vi "MEDIDA_cRIO_ZNB_AMI.vi"(8 "error in (no error)":errorcluster) -> (0 "error out":errorcluster)   [LabVIEW 2017]
uses:
  MEDIDA_cRIO_ZNB_AMI_DATOS.ctl
  MEDIDA_cRIO_ZNB_AMI.ctl
  RohdeSchwarz ZNB MeasConfig.ctl
  AMI MAGNET/Status AMI.ctl
  DISPLAY/Display_Command Control.ctl
  DISPLAY/DataType.ctl
  TIMING/Timing_Module Control.ctl
  cRIO_ZNB_AMI_GLOBALES.vi
  FILE/File_Module Control.ctl
  <instrlib>/Agilent ENA Series/Agilent ENA Series.lvlib
panel:
  out "Z.Stable":bool
  out "Y.Stable":bool
  out "X.Stable":bool
  out "wZ.Stable":bool
  out "wY.Stable":bool
  out "wX.Stable":bool
  out "Z.WaitStability":bool
  out "Y.WaitStability":bool
  out "X.WaitStability":bool
  out "X state":T1=1 items=["Unknown", "RAMPING to target field/current", "HOLDING at the target field/current", "PAUSED", "Ramping in MANUAL UP mode", "Ramping in MANUAL DOWN mode", "ZEROING CURRENT (in progress)", "Quench detected", "At ZERO current", "Heating persistent switch", "Cooling persistent switch", "External Rampdown active"]
  out "Y state":T1=1 items=["Unknown", "RAMPING to target field/current", "HOLDING at the target field/current", "PAUSED", "Ramping in MANUAL UP mode", "Ramping in MANUAL DOWN mode", "ZEROING CURRENT (in progress)", "Quench detected", "At ZERO current", "Heating persistent switch", "Cooling persistent switch", "External Rampdown active"]
  out "Z state":T1=1 items=["Unknown", "RAMPING to target field/current", "HOLDING at the target field/current", "PAUSED", "Ramping in MANUAL UP mode", "Ramping in MANUAL DOWN mode", "ZEROING CURRENT (in progress)", "Quench detected", "At ZERO current", "Heating persistent switch", "Cooling persistent switch", "External Rampdown active"]
  out "Z Modo Rampa":u16(ring)=1 items=["RAMP", "PAUSE", "PAUSE", "MANUAL DOWN", "ZERO"]
  out "Z Rate":dbl
  out "Z Field":dbl
  out "Y Modo Rampa":u16(ring)=1 items=["RAMP", "PAUSE", "PAUSE", "MANUAL DOWN", "ZERO"]
  out "Y Rate":dbl
  out "Y Field":dbl
  out "X Modo Rampa":u16(ring)=1 items=["RAMP", "PAUSE", "PAUSE", "MANUAL DOWN", "ZERO"]
  out "X Rate":dbl
  out "X Field":dbl
  in  "ID Query? (T: Yes)":bool=TRUE
  in  "Reset? (T: Yes)":bool
  out "XY lastMeas":cluster{dbl[], dbl[]}(graph)
  in  "VISA resource":refnum<visa-resource-name>="ZNB20-62-101710"
  out "ENA3G path":path caption="selected path"
  out "MeasConfig":T2={"Tiempo (sec)"=10.0, "Campo X (T)"=0.025, "Campo Y (T)"=10.0, "Campo Z (T)"=0.025, "Temperatura (K)"=0.025, "Start Frequency (Hz)"=100000.0, "Stop Frequency (Hz)"=1000000.0, "IF Bandwidth"=25.0, "Sweep time(s)"=25.0, "Meas Points"=201, "Power Level (0.0)"=-40.0} {"Campo Z (T)" format="%^.2e"; "Campo Y (T)" format="%^.2e"; "Sweep time(s)" format="%^.2g"; "Temperatura (K)" format="%^.2e"; "Campo X (T)" format="%^.2e"; "Tiempo (sec)" format="%^.2g"; "Start Frequency (Hz)" format="%^.2e"; "IF Bandwidth" format="%^.2e"; "Power Level (0.0)" format="%^.2g"}
  out "Voltage Status":i32(ring) items=["VoltageUnknown", "Stable", "Tracking"]
  out "wV.Stable":bool
  out "V.Stable":bool
  out "V.WaitStability":bool
  out "Command":T3
  out "T.Stable":bool
  out "#seconds":dbl=300.0
  out "currentPoint":i16=300
  out "dSeconds":dbl=300.0
  out "averages":i16=300
  out "#points":i16=300
  out "On timeout":i32(ring) items=["Continue", "Abort "]
  out "StabilityTimeout(s)":dbl=300.0
  out "wT.Stable":bool
  out "T.WaitStability":bool
  out "#IntruccionActual":i32
  out "#Intrucciones":i32
  out "Temperature Status":i32(ring) items=["TemperatureUnknown", "Stable", "Tracking", "Near"]
  out "cRIO Stable":bool
  out "Datos":T4 {"CampoZ(T)" format="%.3e"; "CampoY(T)" format="%.3e"; "A.Input3(V)" format="%.3e"; "A.Input4(V)" format="%.3e"; "A.Input1(V)" format="%.3e"; "A.Input2(V)" format="%.3e"; "Temperatura(K)" format="%.3e"; "CampoX(T)" format="%.3e"; "Tiempo(min)" format="%.3e"}
  # "cRIO"
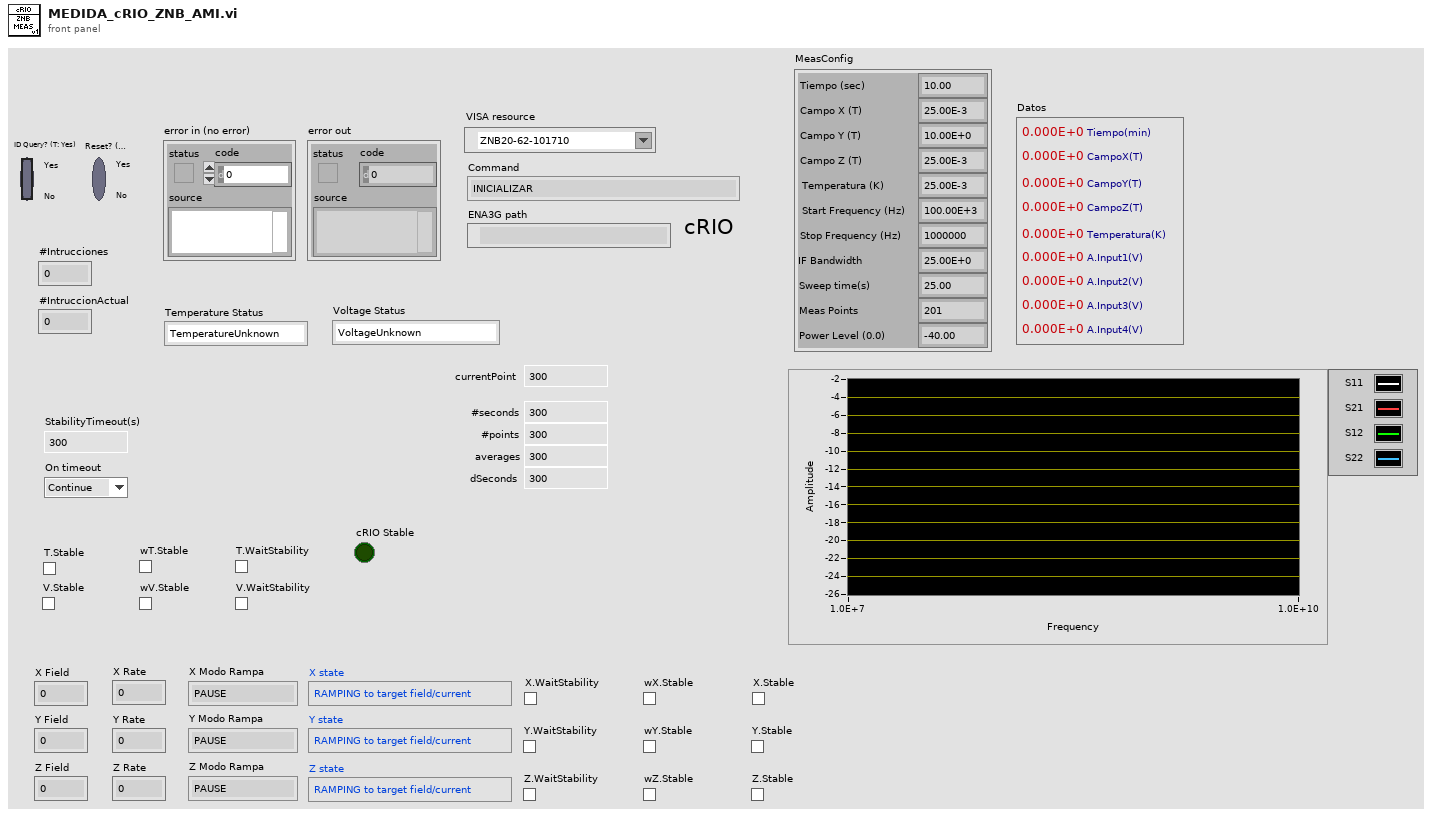
[diagram p1: front panel]
types:
  T1 = typedef "Status AMI.ctl" = u16
  T2 = typedef "RohdeSchwarz ZNB MeasConfig.ctl" = cluster{"Tiempo (sec)":dbl, "Campo X (T)":dbl, "Campo Y (T)":dbl, "Campo Z (T)":dbl, "Temperatura (K)":dbl, "Start Frequency (Hz)":dbl, "Stop Frequency (Hz)":dbl, "IF Bandwidth":dbl, "Sweep time(s)":dbl, "Meas Points":i32, "Power Level (0.0)":dbl}
  T3 = typedef "MEDIDA_cRIO_ZNB_AMI.ctl" = enum16{"INICIALIZAR", "TEST COMMAND", "SET FIELD X", "LOOK STABLE FIELD X", "SET FIELD Y", "LOOK STABLE FIELD Y", "SET FIELD Z", "LOOK STABLE FIELD Z", "SET TEMPERATURE", "LOOK STABLE TEMPERATURE", "SET VOLTAGE", "LOOK STABLE VOLTAGE", "WAIT PARAMETERS", "LOOK STABILITY", "MEASURE PARAMETERS", "SCAN READ TIME, B y T", "SCAN READ cRIO", "MEASURE SWEEP", "SWEEP READ TIME, B y T", "SWEEP READ cRIO", "MEASURE ENA3G / ZNB", "PAUSE SEQUENCE", "FINALIZAR"}
  T4 = typedef "MEDIDA_cRIO_ZNB_AMI_DATOS.ctl" = cluster{"Tiempo(min)":dbl, "CampoX(T)":dbl, "CampoY(T)":dbl, "CampoZ(T)":dbl, "Temperatura(K)":dbl, "A.Input1(V)":dbl, "A.Input2(V)":dbl, "A.Input3(V)":dbl, "A.Input4(V)":dbl}
  T5 = typedef "DataType.ctl" = enum16{"Initialize Front Panel", "Update Front Panel", "Update Graph", "Enable/Disable Controls", "Update Status"}
  T6 = typedef "Display_Command Control.ctl" = enum16{"Initialize", "Generate Event", "Shutdown"}
  T7 = enum16{"open", "replace", "create", "open or create", "replace or create", "replace or create with confirmation"}
  T8 = typedef "Timing_Module Control.ctl" = enum16{"Initialize Time", "Check Time"}
  T9 = typedef "File_Module Control.ctl" = enum16{"Initialize", "Save Head", "Save Data", "Shutdown"}
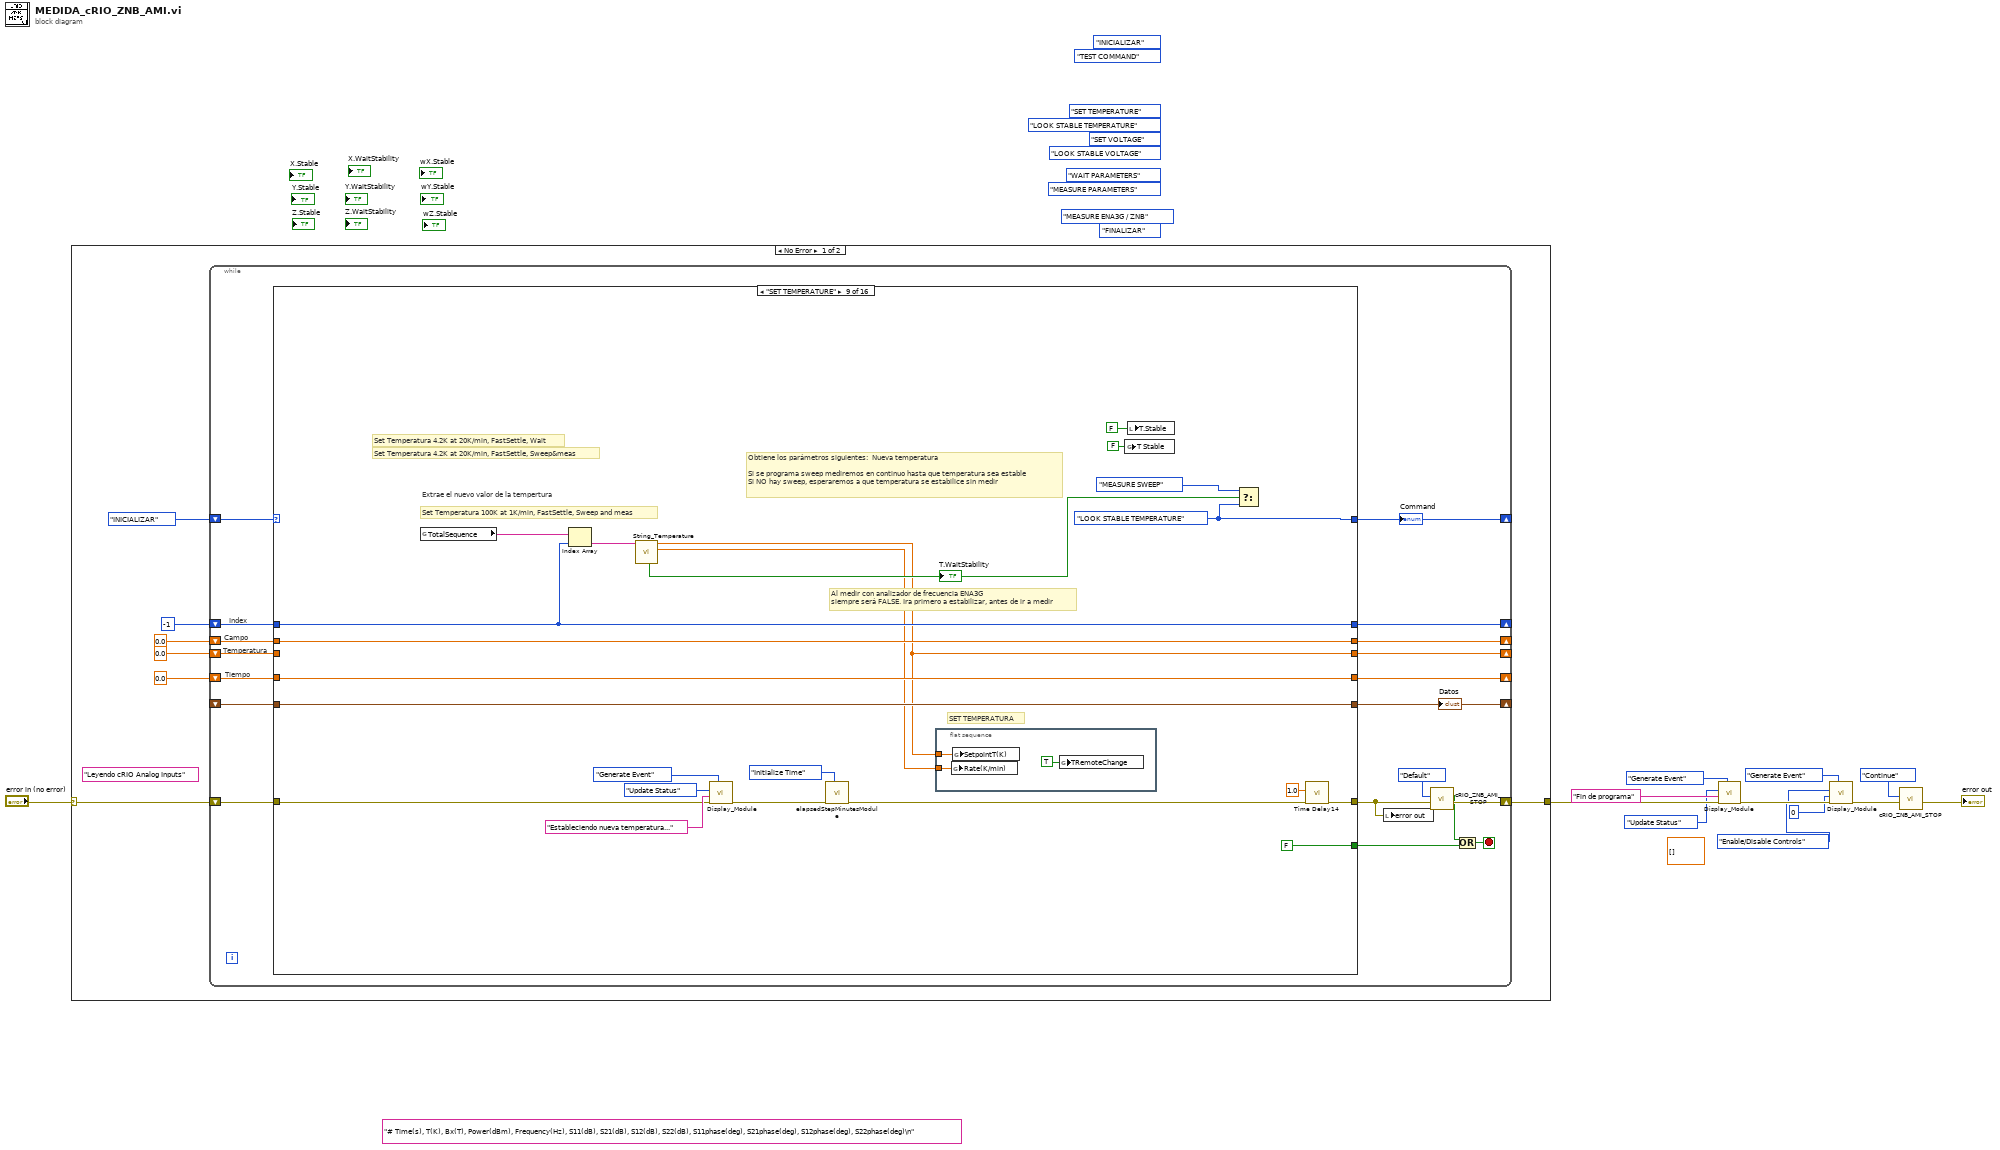
[diagram p0: block diagram]
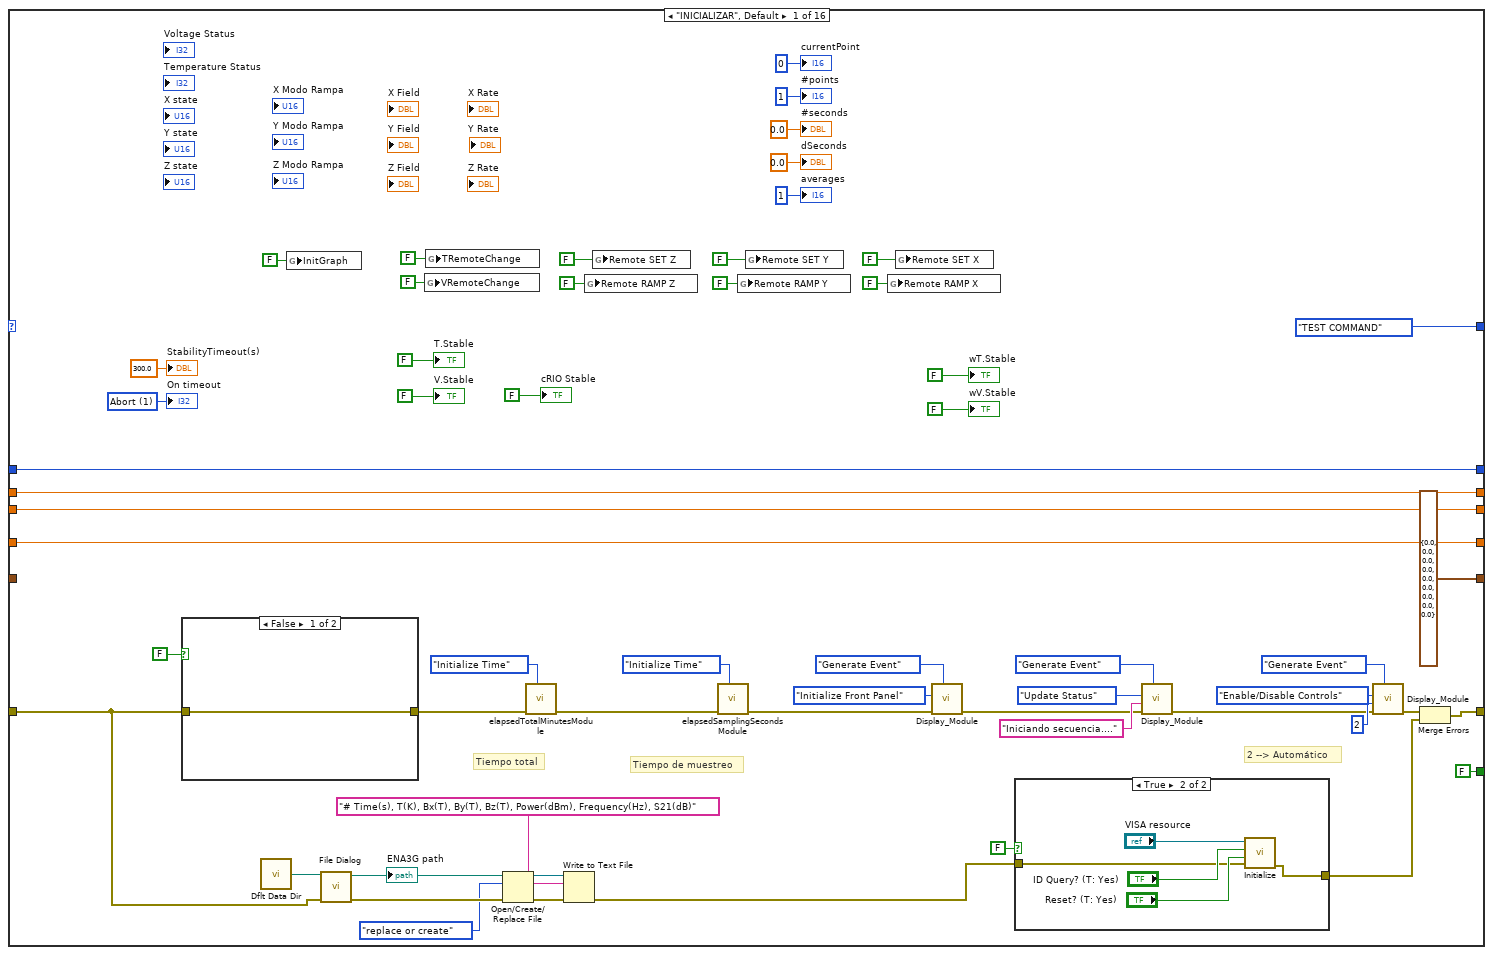
[diagram p2: hidden frame]
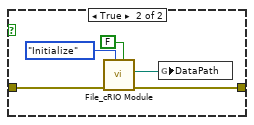
[diagram p4: hidden frame]
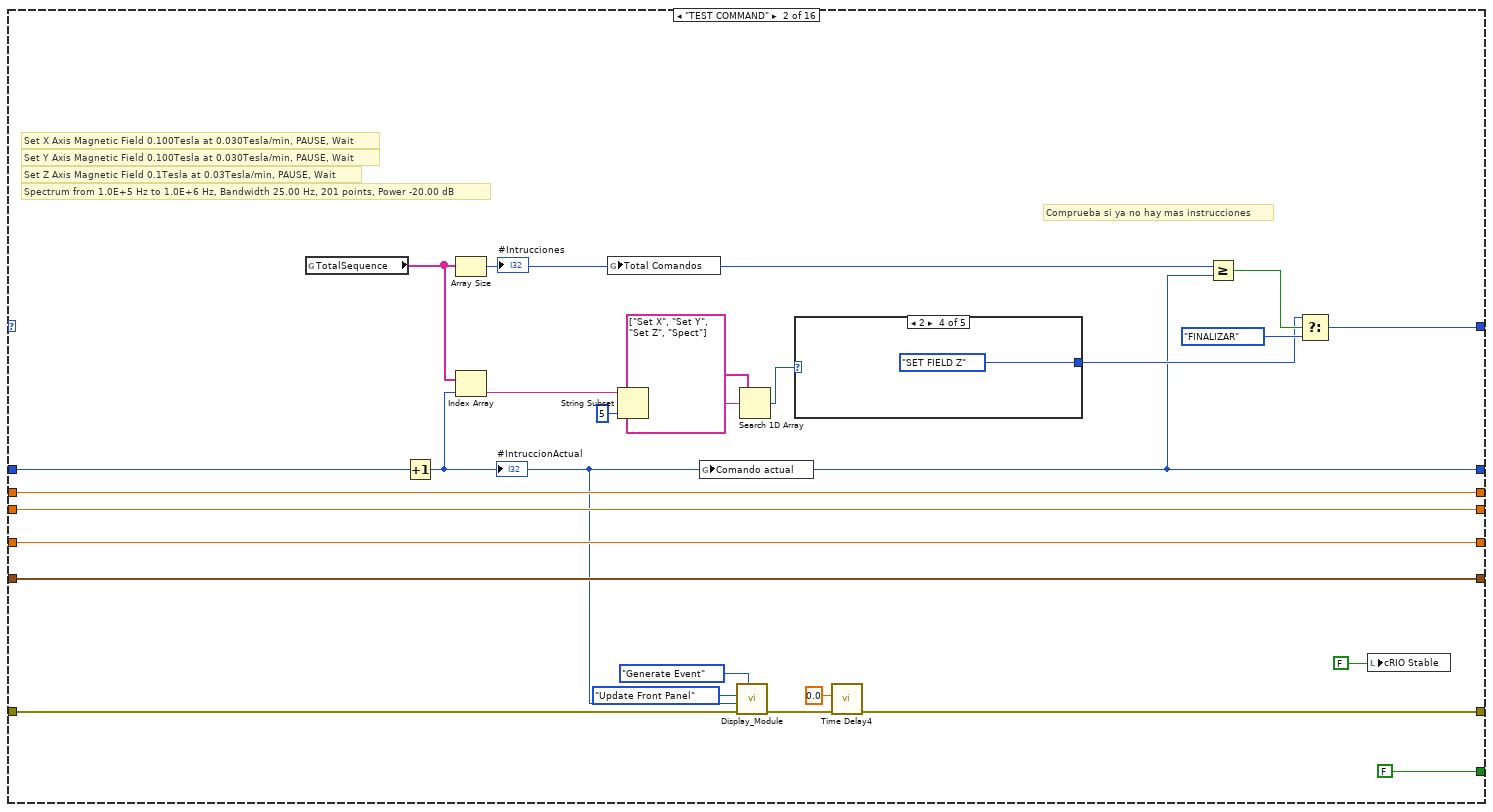
[diagram p5: hidden frame]
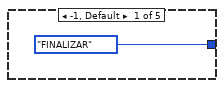
[diagram p6: hidden frame]
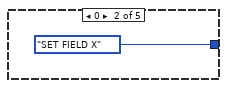
[diagram p7: hidden frame]
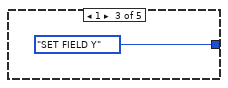
[diagram p8: hidden frame]
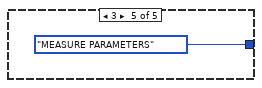
[diagram p9: hidden frame]
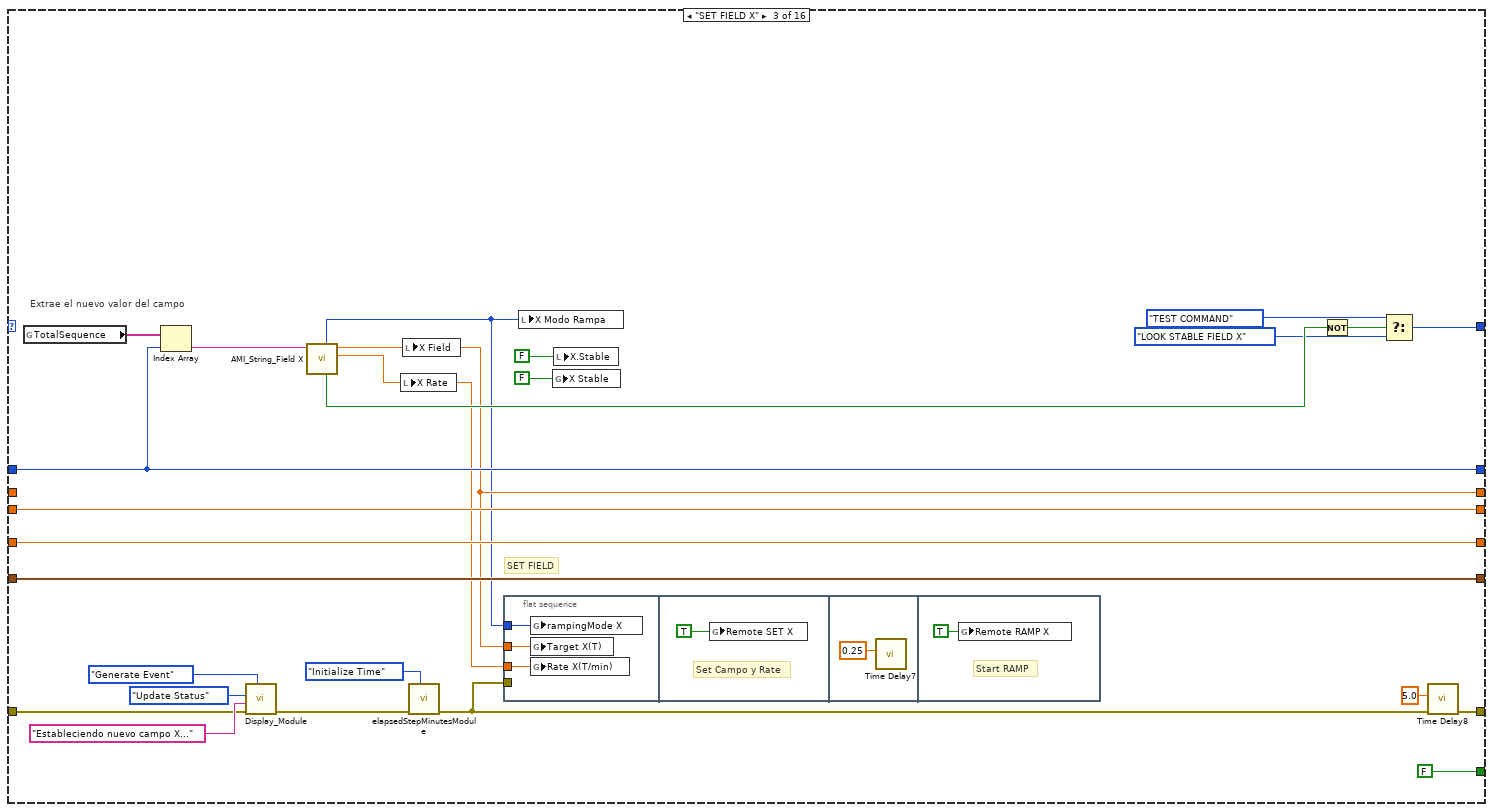
[diagram p10: hidden frame]
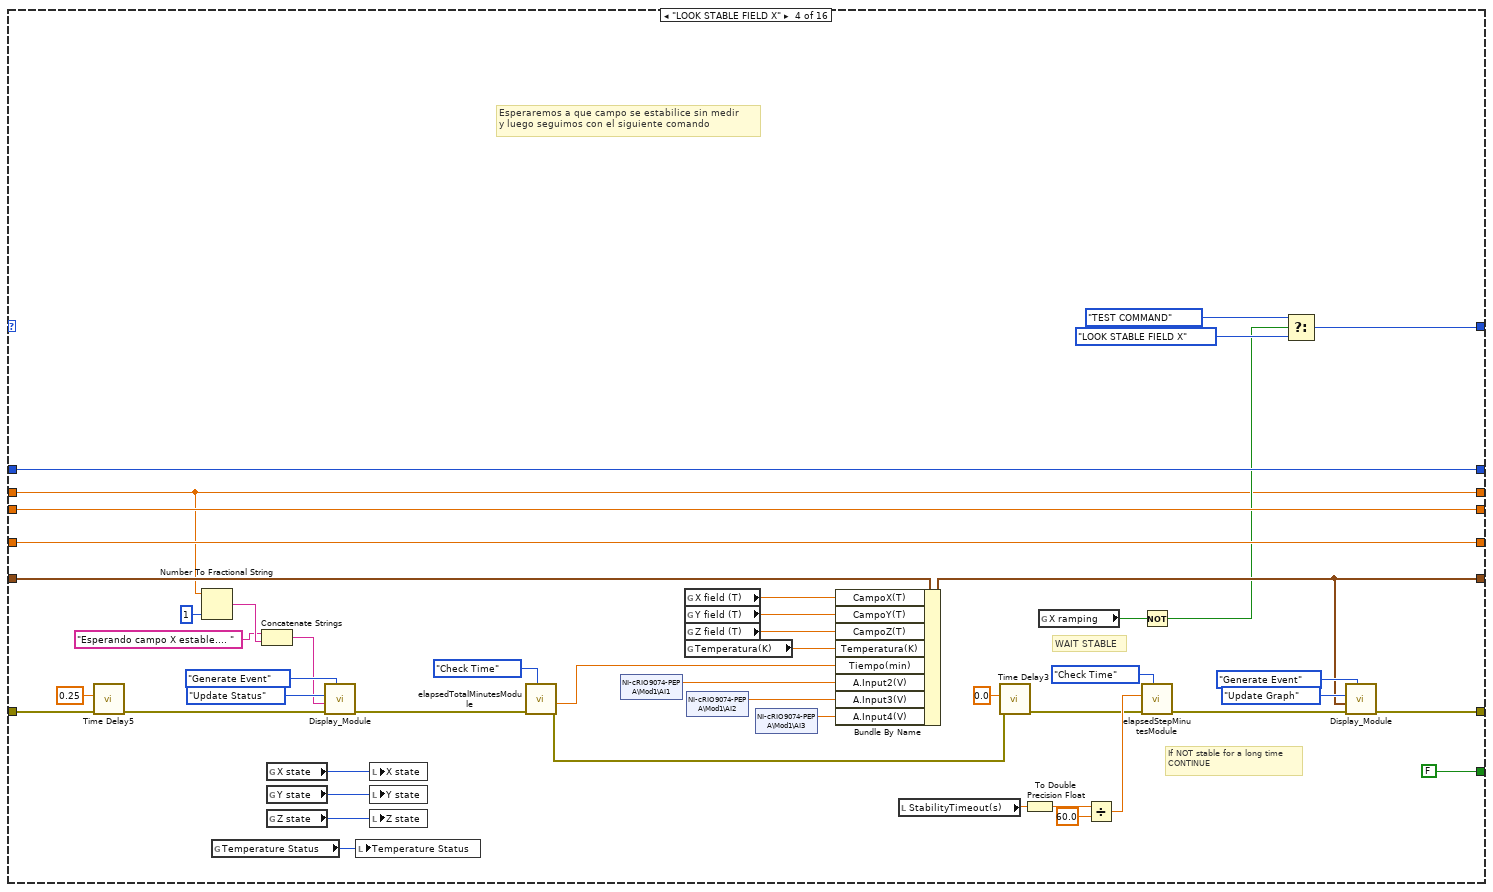
[diagram p11: hidden frame]
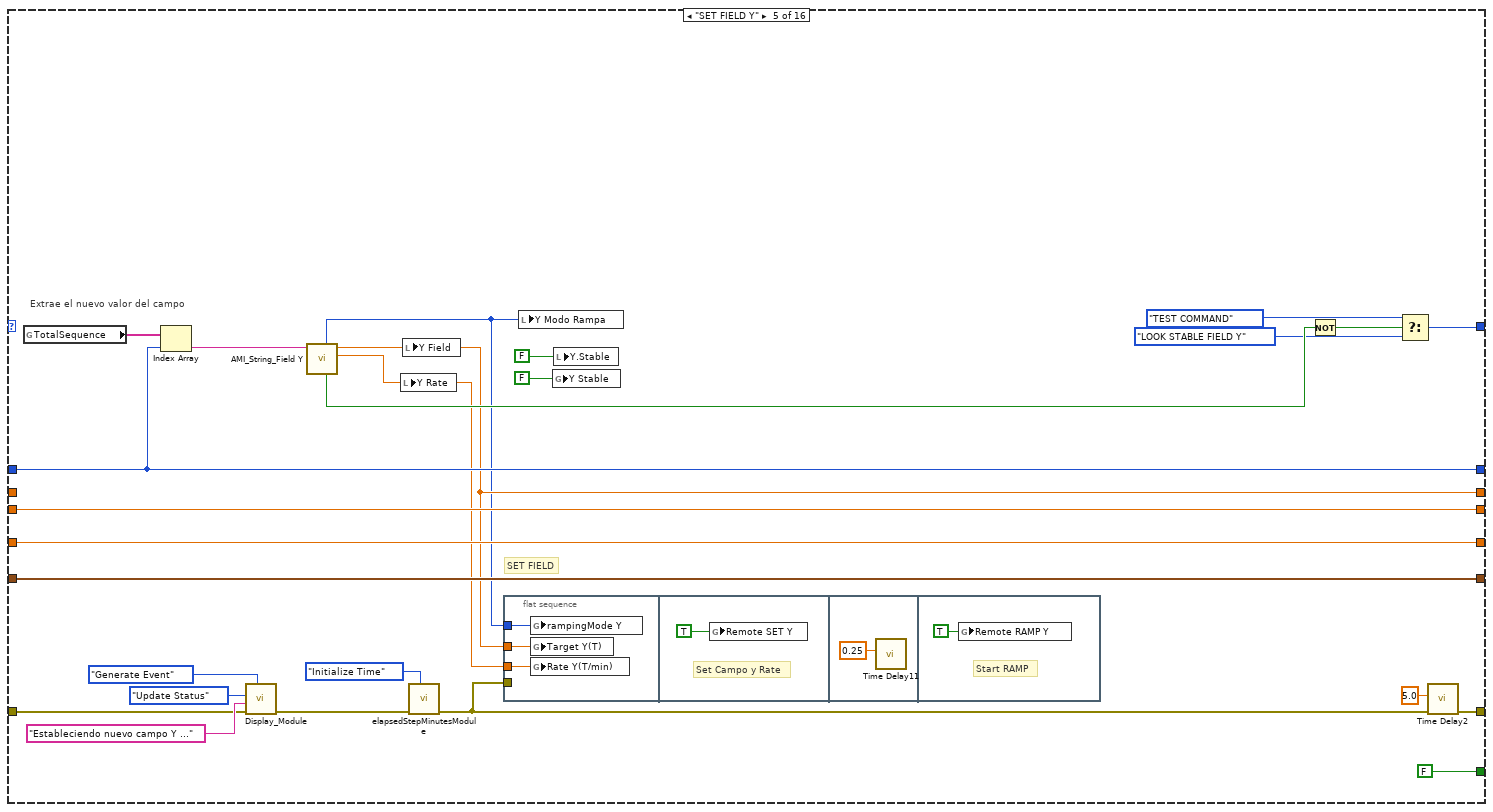
[diagram p12: hidden frame]
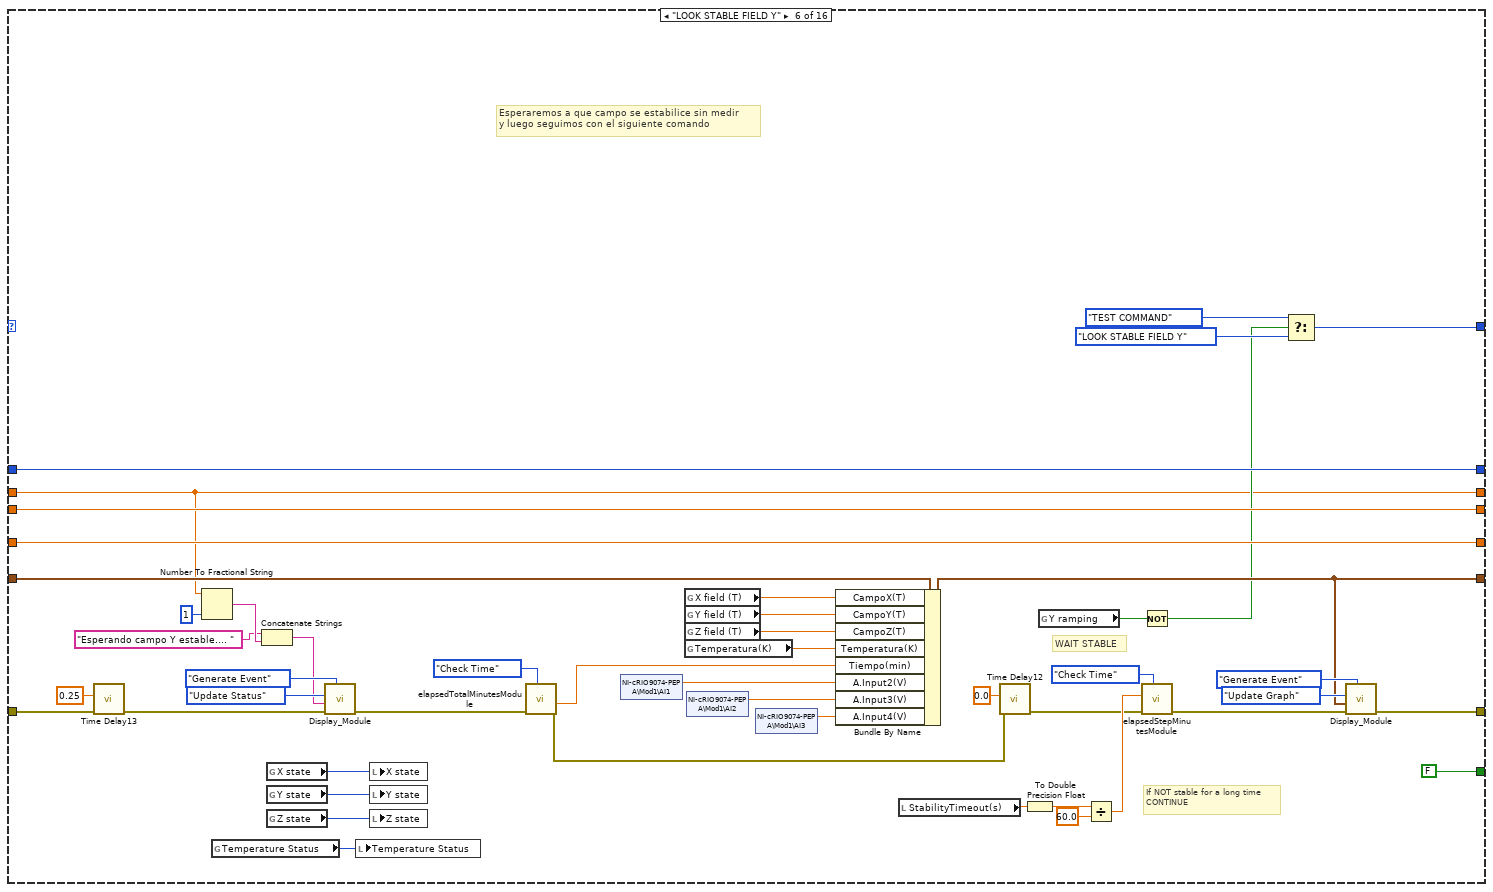
[diagram p13: hidden frame]
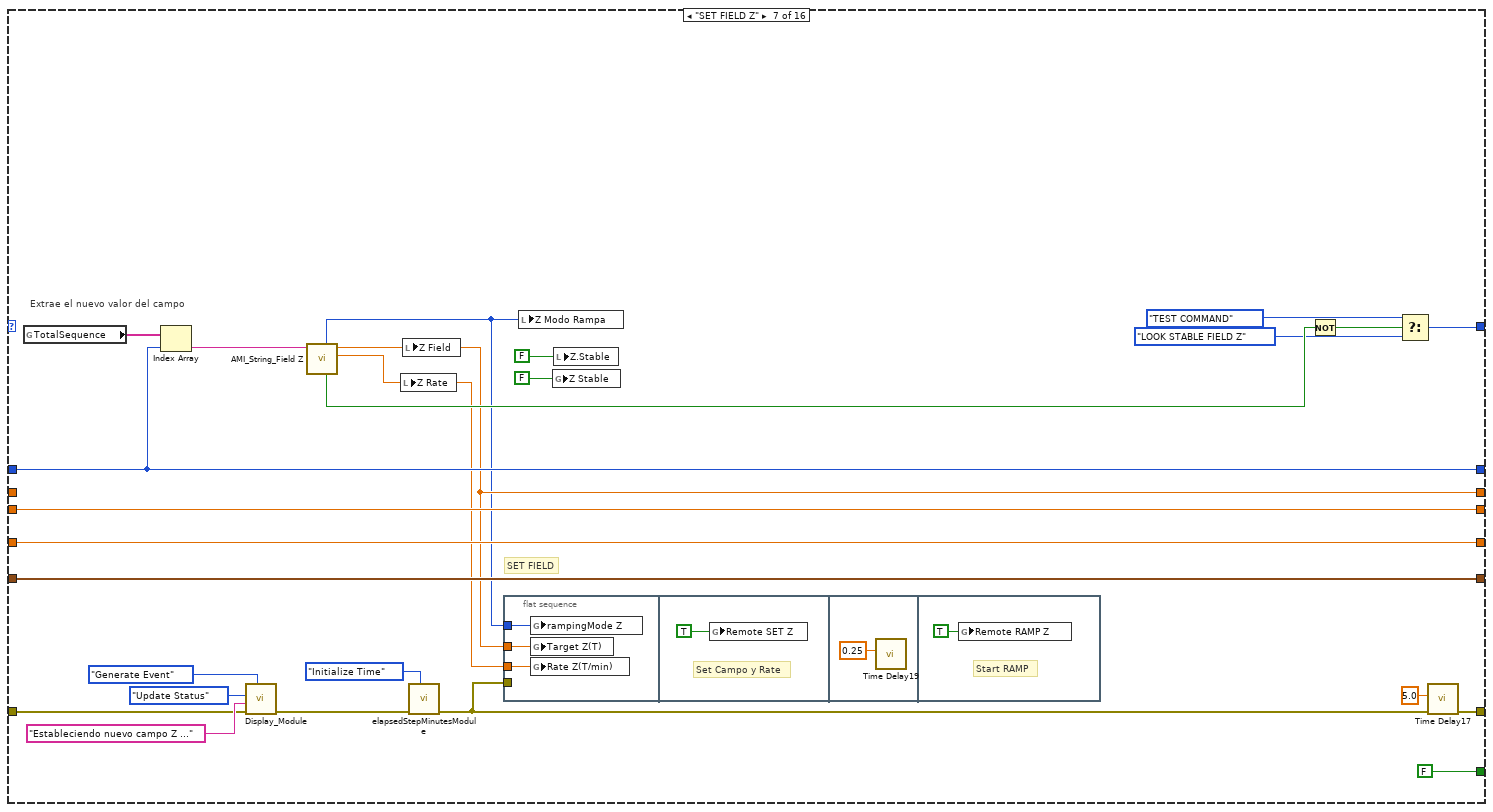
[diagram p14: hidden frame]
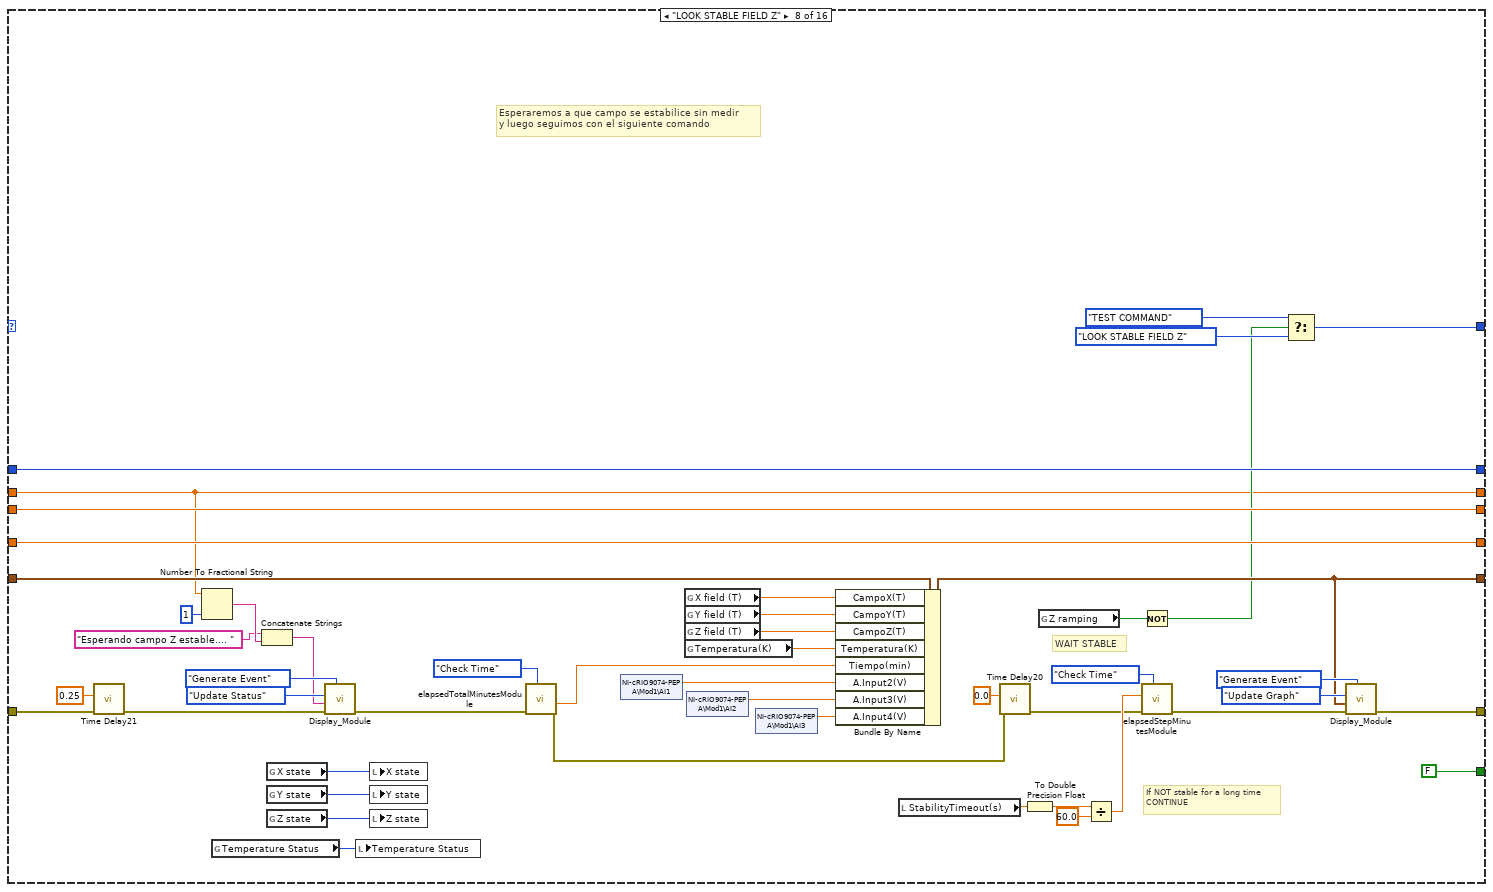
[diagram p15: hidden frame]
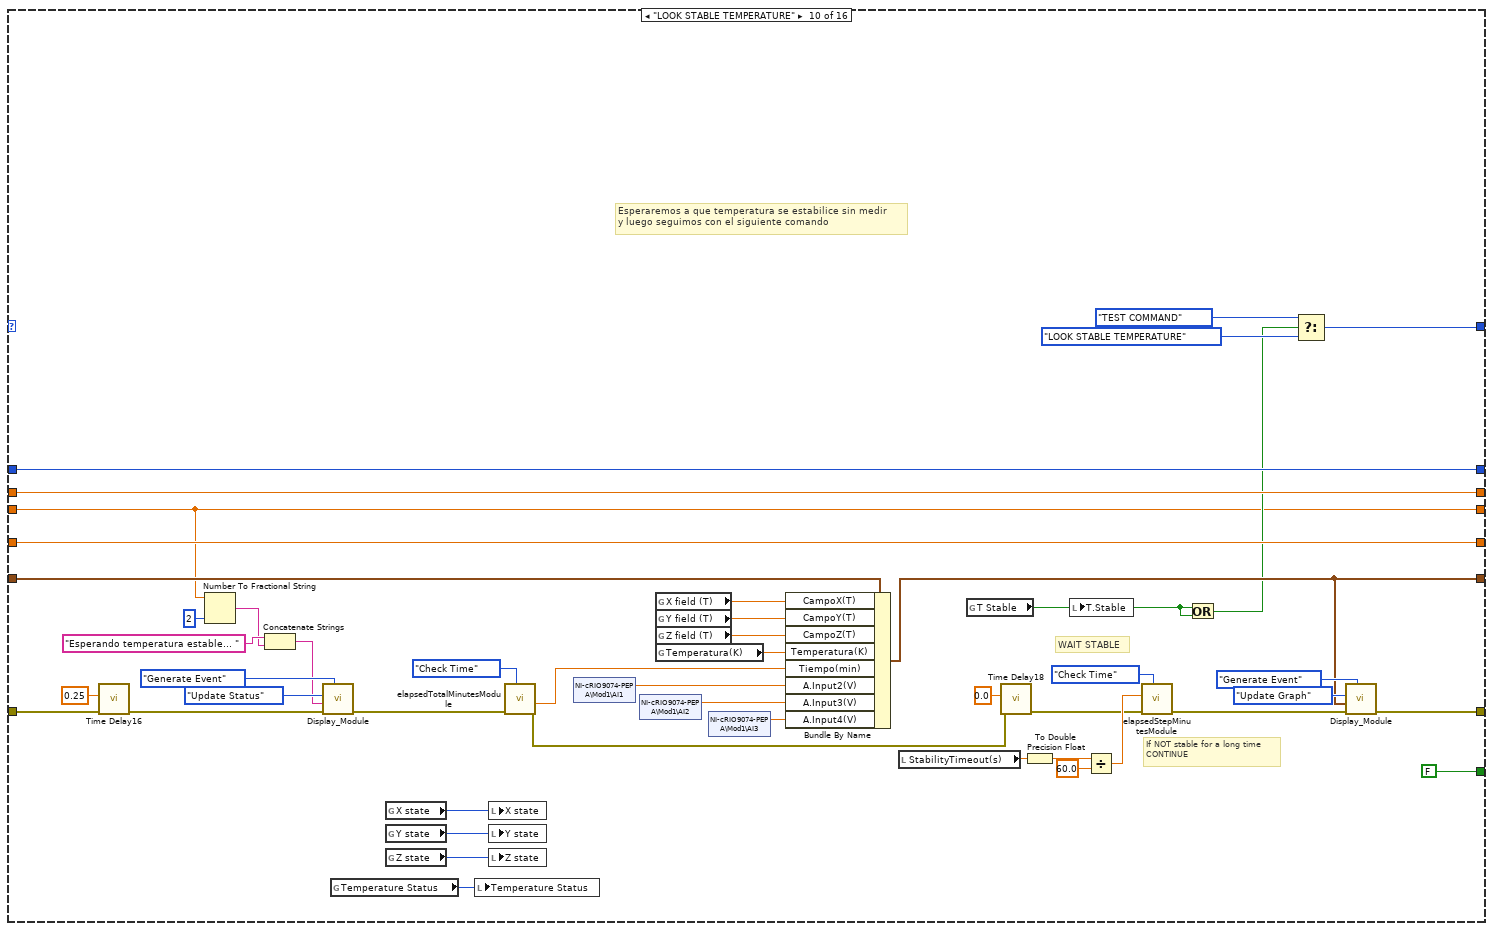
[diagram p16: hidden frame]
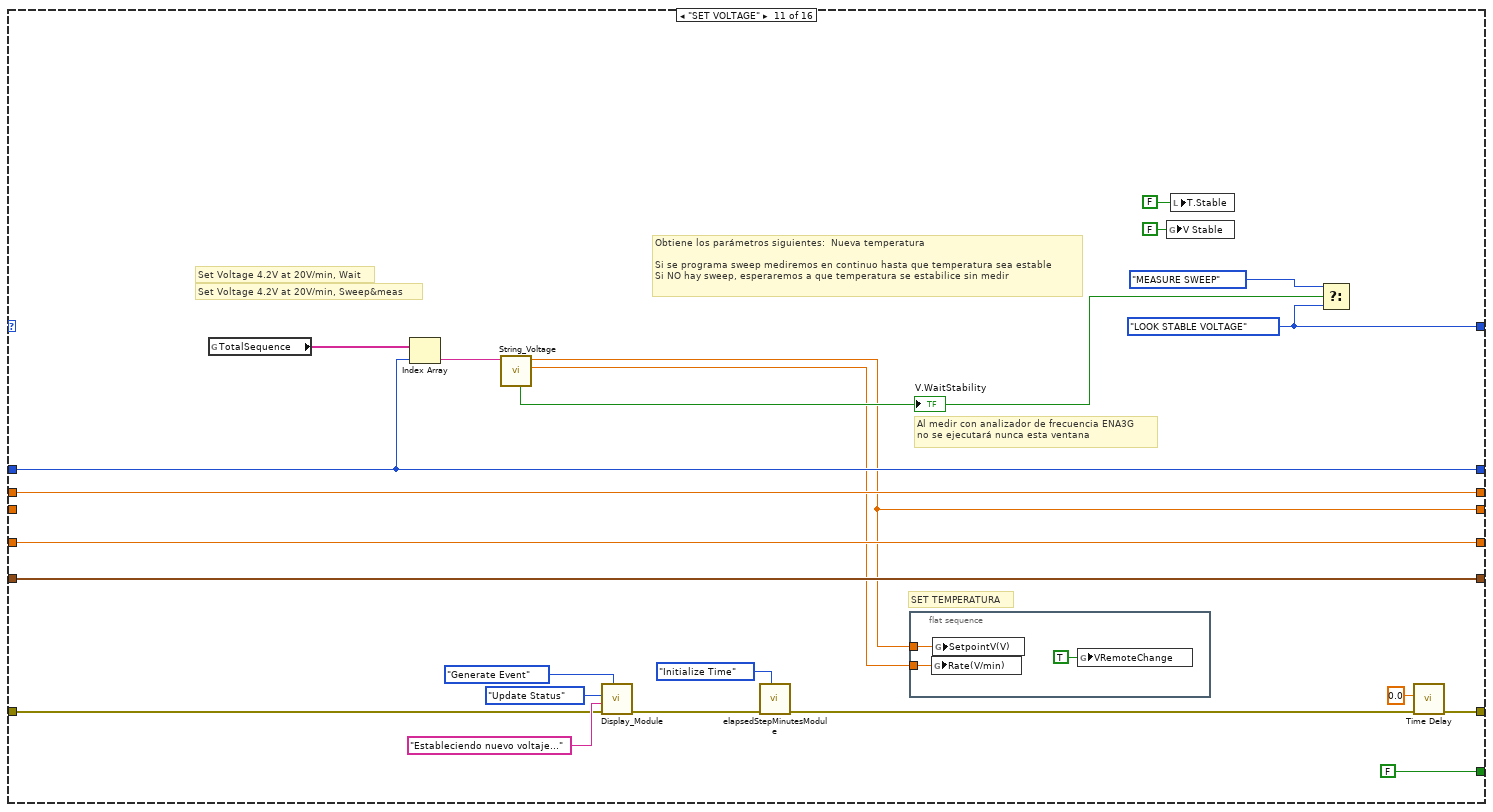
[diagram p17: hidden frame]
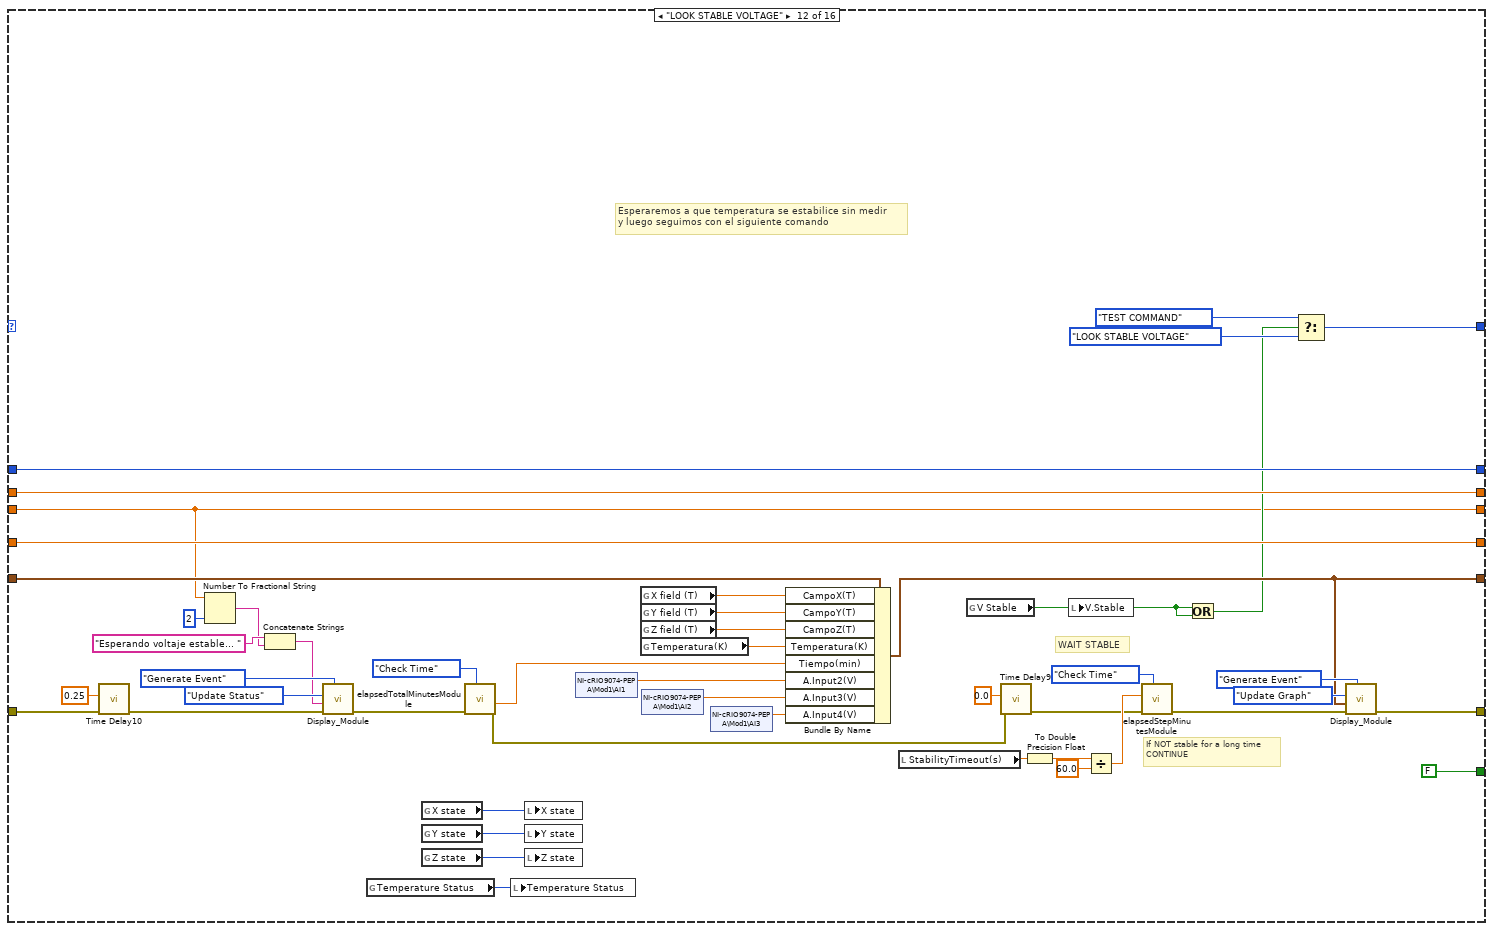
[diagram p18: hidden frame]
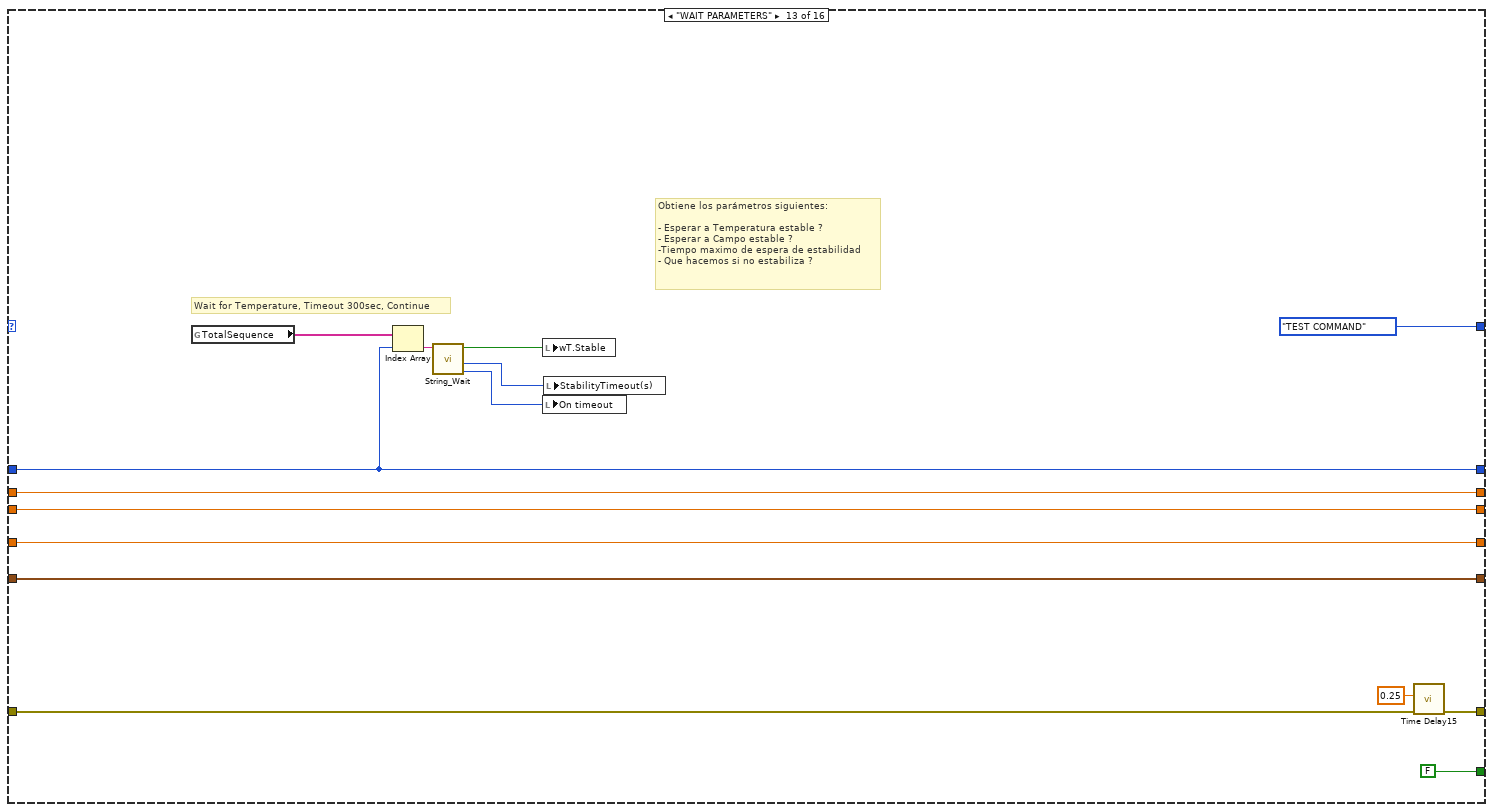
[diagram p19: hidden frame]
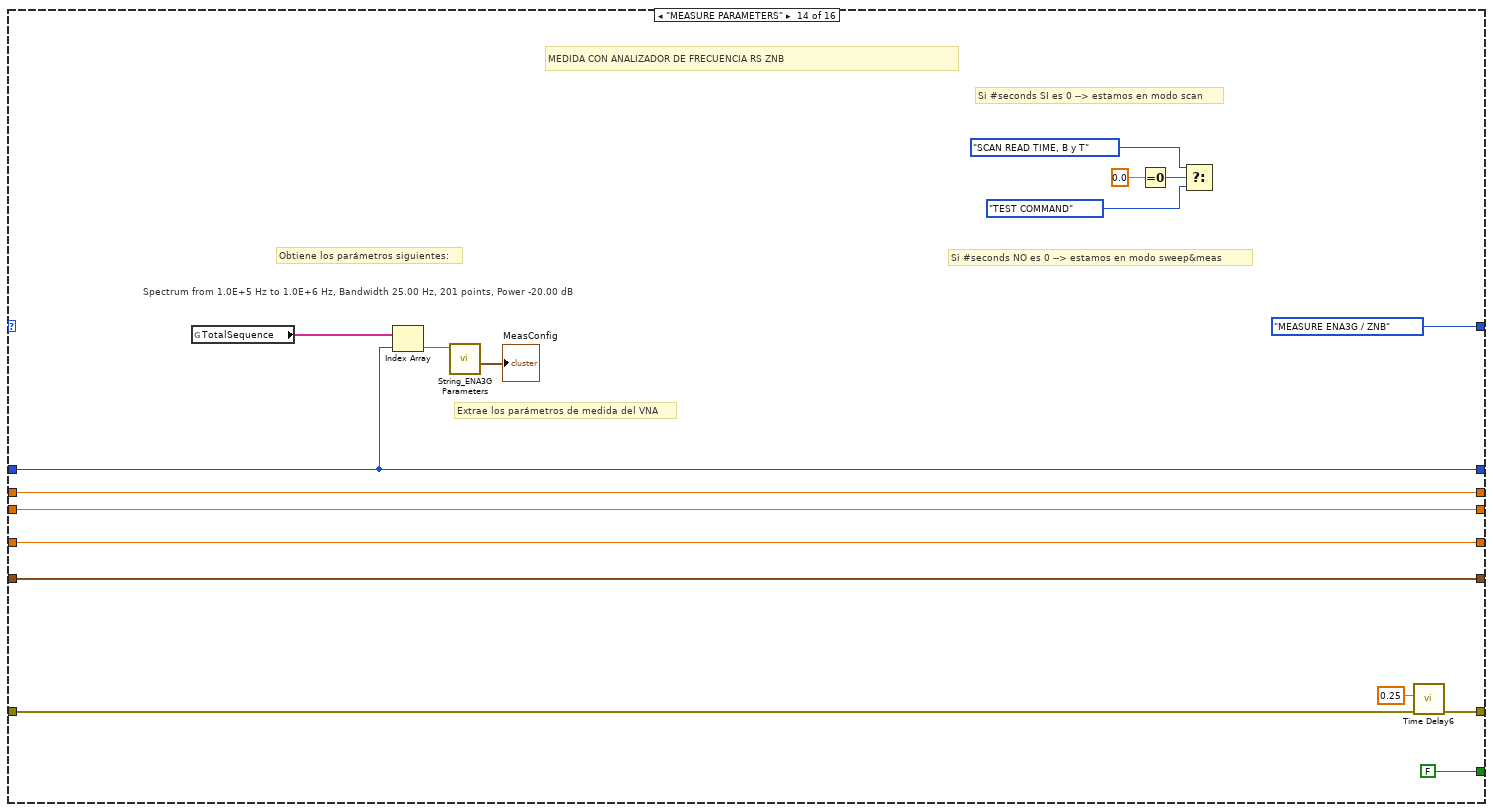
[diagram p20: hidden frame]
diagram:
  (unwired) "# Time(s), T(K), Bx(T), Power(dBm), Frequency(Hz), S11(dB), S21(dB), S12(dB), S22(dB), S11phase(deg), S21phase(deg), S12phase(deg), S22phase(deg)\n" ("format string")
  (unwired) MEDIDA_cRIO_ZNB_AMI."TEST COMMAND" ("Command")
  (unwired) MEDIDA_cRIO_ZNB_AMI."INICIALIZAR" ("Command")
  (unwired) MEDIDA_cRIO_ZNB_AMI."FINALIZAR" ("Command")
  (unwired) MEDIDA_cRIO_ZNB_AMI."MEASURE ENA3G / ZNB" ("Command")
  (unwired) MEDIDA_cRIO_ZNB_AMI."MEASURE PARAMETERS" ("Command")
  (unwired) MEDIDA_cRIO_ZNB_AMI."WAIT PARAMETERS" ("Command")
  (unwired) MEDIDA_cRIO_ZNB_AMI."LOOK STABLE VOLTAGE" ("Command")
  (unwired) MEDIDA_cRIO_ZNB_AMI."SET VOLTAGE" ("Command")
  (unwired) MEDIDA_cRIO_ZNB_AMI."LOOK STABLE TEMPERATURE" ("Command")
  (unwired) MEDIDA_cRIO_ZNB_AMI."SET TEMPERATURE" ("Command")
  (unwired) dbl[][] [] ("Intensity Graph")
  n1 = case shown="No Error" "error in (no error)" {
    selector: "error in (no error)" -> [w19 w605]
    tunnel: [w18 w605] -> w6
    frame No Error {
      (unwired) "Leyendo cRIO Analog Inputs"
      n2 = while {
        shift-right: [w31] -> _
        shift-left: MEDIDA_cRIO_ZNB_AMI."INICIALIZAR" ("Command") -> [w35]
        shift-right: [w34] -> w18
        shift-left: w19 -> [w36]
        shift-right: [w23] -> _
        shift-left: _ -> [w30]
        shift-right: [w28] -> _
        shift-left: -1 ("milliseconds to wait") -> [w29]
        shift-right: [w25] -> _
        shift-left: 0.0 -> [w26]
        shift-right: [w24] -> _
        shift-left: 0.0 -> [w27]
        shift-right: [w21] -> _
        shift-left: 0.0 -> [w22]
        stop <- w38 stop-if-true
        # "Tiempo"
        # "Temperatura"
        # "Index"
        # "Campo"
        n3 = case shown="\"SET TEMPERATURE\"" w35 {
          tunnel: [FALSE FALSE FALSE FALSE FALSE FALSE FALSE FALSE FALSE FALSE FALSE FALSE FALSE FALSE FALSE TRUE] -> w37
          tunnel: w36 -> [w52 w116 w151 w193 w230 w272 w309 w351 w386 w426 w459 w499 w524 w542 w577 w589]
          tunnel: [w49 w114 w159 w195 w238 w274 w317 w353 w394 w424 w467 w497 w531 w548 w568 w590] -> w20
          tunnel: [MEDIDA_cRIO_ZNB_AMI."TEST COMMAND" ("Command") w128 w140 w208 w219 w287 w298 w366 w375 w439 w448 w512 MEDIDA_cRIO_ZNB_AMI."TEST COMMAND" ("Command") MEDIDA_cRIO_ZNB_AMI."MEASURE ENA3G / ZNB" ("Command") MEDIDA_cRIO_ZNB_AMI."TEST COMMAND" ("Command") MEDIDA_cRIO_ZNB_AMI."FINALIZAR" ("Command")] -> w31
          tunnel: [T4 {"Tiempo(min)"=0.0, "CampoX(T)"=0.0, "CampoY(T)"=0.0, "CampoZ(T)"=0.0, "Temperatura(K)"=0.0, "A.Input1(V)"=0.0, "A.Input2(V)"=0.0, "A.Input3(V)"=0.0, "A.Input4(V)"=0.0} ("Datos") w131 w162 w202 w241 w281 w320 w360 w396 w433 w469 w506 w534 w551 w586 w602] -> w23
          tunnel: w30 -> [_ w131 w162 w203 w241 w282 w320 w361 w396 w434 w469 w507 w534 w551 w587 w602]
          tunnel: w29 -> [w91 w121 w163 w214 w242 w293 w321 w372 w397 w445 w470 w518 w535 w552 w582 w601]
          tunnel: [w91 w109 w163 w214 w242 w293 w321 w372 w397 w445 w470 w518 w535 w552 w582 w601] -> w28
          tunnel: w27 -> [w89 w117 w160 w212 w239 w291 w318 w370 _ w419 _ w492 w532 w549 w584 w592]
          tunnel: w26 -> [w90 w118 _ w187 _ w266 _ w345 w380 w443 w453 w516 w525 w543 w583 w593]
          tunnel: [w90 w118 w143 w187 w222 w266 w301 w345 w380 w443 w453 w516 w525 w543 w583 w593] -> w25
          tunnel: [w89 w117 w160 w212 w239 w291 w318 w370 w378 w419 w451 w492 w532 w549 w584 w592] -> w24
          tunnel: w22 -> [w80 w113 w158 w207 w237 w286 w316 w365 w393 w438 w466 w511 w530 w547 w585 w591]
          tunnel: [w80 w113 w158 w207 w237 w286 w316 w365 w393 w438 w466 w511 w530 w547 w585 w591] -> w21
          frame "INICIALIZAR", Default {
            w74 = 1 items=["Continue", "Abort "] ("On timeout")
            # "Tiempo de muestreo"
            # "Tiempo total"
            # "2 --> Automático"
            n4 = case shown="False" FALSE {
              tunnel: w52 -> [w102 w106]
              tunnel: [w102 w105] -> w66
              frame False {
              }
              frame True {
                n5 = call "File_cRIO Module.vi"("Estado"=FALSE, "Command"=File_Module_Control."Initialize", "error in (no error)"=w106) -> ("error out"=w105:errorcluster, "selected path"=w103:path)  [unwired: 7 in]
                n6 = global write "cRIO_ZNB_AMI_GLOBALES.vi" "DataPath"(w103) -> ()
              }
            }
            n7 = call <vilib>:"Dflt Data Dir.vi"() -> ("App:Default Data Directory"=w56:path)
            n8 = global write "cRIO_ZNB_AMI_GLOBALES.vi" "InitGraph"(FALSE ("InitGraph")) -> ()
            n9 = call "File Dialog"("start path"=w56, "error in"=w52) -> ("selected path"=w55:path, "error out"=w54:errorcluster)  [unwired: 10 in, 2 out]
            "ENA3G path" <- w55
            n10 = global write "cRIO_ZNB_AMI_GLOBALES.vi" "VRemoteChange"(FALSE ("TRemoteChange")) -> ()
            n11 = global write "cRIO_ZNB_AMI_GLOBALES.vi" "TRemoteChange"(FALSE ("TRemoteChange")) -> ()
            n12 = Open/Create/Replace File(file path (use dialog)=w55, error in=w54, operation (0:open)=T7."replace or create") -> (refnum out=w57:refnum<file>, error out=w51:errorcluster)  [unwired: 3 in, 1 out]
            n13 = call "elapsedTotalMinutesModule.vi"("Command"=Timing_Module_Control."Initialize Time", "error in (no error)"=w66) -> ("error out"=w79:errorcluster)  [unwired: 7 in, 2 out]
            n14 = Write to Text File(file (use dialog)=w57, text="# Time(s), T(K), Bx(T), By(T), Bz(T), Power(dBm), Frequency(Hz), S21(dB)" ("format string"), error in=w51) -> (error out=w48:errorcluster)  [unwired: 1 in, 2 out]
            n15 = global write "cRIO_ZNB_AMI_GLOBALES.vi" "Remote RAMP Z"(FALSE ("TRemoteChange")) -> ()
            n16 = global write "cRIO_ZNB_AMI_GLOBALES.vi" "Remote SET Z"(FALSE ("TRemoteChange")) -> ()
            n17 = call "elapsedSamplingSecondsModule.vi"("Command"=Timing_Module_Control."Initialize Time", "error in (no error)"=w79) -> ("error out"=w78:errorcluster)  [unwired: 7 in, 2 out]
            n18 = global write "cRIO_ZNB_AMI_GLOBALES.vi" "Remote RAMP Y"(FALSE ("TRemoteChange")) -> ()
            n19 = global write "cRIO_ZNB_AMI_GLOBALES.vi" "Remote SET Y"(FALSE ("TRemoteChange")) -> ()
            n20 = global write "cRIO_ZNB_AMI_GLOBALES.vi" "Remote RAMP X"(FALSE ("TRemoteChange")) -> ()
            n21 = global write "cRIO_ZNB_AMI_GLOBALES.vi" "Remote SET X"(FALSE ("TRemoteChange")) -> ()
            n22 = call "Display_Module.vi"("Command"=Display_Command_Control."Generate Event", "error in (no error)"=w78, "Data Type"=DataType."Initialize Front Panel") -> ("error out"=w82:errorcluster)  [unwired: 8 in]
            n23 = case shown="True" FALSE {
              tunnel: w48 -> [w96 w98]
              tunnel: [w96 w97] -> w47
              frame False {
              }
              frame True {
                n24 = call <instrlib>:"Initialize.vi"("error in (no error)"=w98, "Reset? (T: Yes)"="Reset? (T: Yes)", "ID Query? (T: Yes)"="ID Query? (T: Yes)", "VISA resource name"="VISA resource") -> ("error out"=w97:errorcluster)  [unwired: 6 in, 1 out]
              }
            }
            n25 = call "Display_Module.vi"("Command"=Display_Command_Control."Generate Event", "error in (no error)"=w82, "Data"="Iniciando secuencia...." ("element"), "Data Type"=DataType."Update Status") -> ("error out"=w81:errorcluster)  [unwired: 7 in]
            n26 = call "Display_Module.vi"("Command"=Display_Command_Control."Generate Event", "error in (no error)"=w81, "Data"=2, "Data Type"=DataType."Enable/Disable Controls") -> ("error out"=w50:errorcluster)  [unwired: 7 in]
            n27 = Merge Errors(w50, w47) -> (w49:errorcluster)
            "wT.Stable" <- FALSE ("wT.Stable")
            "StabilityTimeout(s)" <- 300.0 ("StabilityTimeout(s)")
            "On timeout" <- w74
            "cRIO Stable" <- FALSE ("PPMS Stable")
            "#points" <- i16 1 ("points")
            "averages" <- i16 1 ("averages")
            "dSeconds" <- 0.0 ("seconds")
            "currentPoint" <- i16 0 ("point#")
            "#seconds" <- 0.0 ("#seconds")
            "T.Stable" <- FALSE ("T.Stable")
            "V.Stable" <- FALSE ("V.Stable")
            "wV.Stable" <- FALSE ("wV.Stable")
          }
          frame "TEST COMMAND" {
            # "Spectrum from 1.0E+5 Hz to 1.0E+6 Hz, Bandwidth 25.00 Hz, 201 points, Power -20.00 dB"
            # "Set Z Axis Magnetic Field 0.1Tesla at 0.03Tesla/min, PAUSE, Wait"
            # "Set Y Axis Magnetic Field 0.100Tesla at 0.030Tesla/min, PAUSE, Wait"
            # "Set X Axis Magnetic Field 0.100Tesla at 0.030Tesla/min, PAUSE, Wait"
            # "Comprueba si ya no hay mas instrucciones"
            n28 = global read "cRIO_ZNB_AMI_GLOBALES.vi" "TotalSequence"() -> (w111:string[])
            n29 = Increment(x=w121) -> (x+1=w109:i32)
            "#IntruccionActual" <- w109
            n30 = Array Size(array=w111) -> (size(s)=w108:i32)
            "#Intrucciones" <- w108
            n31 = Index Array(array=w111, index=w109) -> (element=w126:string)
            n32 = global write "cRIO_ZNB_AMI_GLOBALES.vi" "Total Comandos"(w108) -> ()
            n33 = String Subset(string=w126, length (rest)=5 ("length (rest)")) -> (substring=w124:string)  [unwired: 1 in]
            n34 = global write "cRIO_ZNB_AMI_GLOBALES.vi" "Comando actual"(w109) -> ()
            n35 = call "Display_Module.vi"("Command"=Display_Command_Control."Generate Event", "error in (no error)"=w116, "Data"=w109, "Data Type"=DataType."Update Front Panel") -> ("error out"=w115:errorcluster)  [unwired: 7 in]
            n36 = Search 1D Array(1D array=string[] ["Set X", "Set Y", "Set Z", "Spect"], element=w124) -> (index of element=w123:i32)  [unwired: 1 in]
            n37 = case shown="2" w123 {
              tunnel: [MEDIDA_cRIO_ZNB_AMI."FINALIZAR" ("Command") MEDIDA_cRIO_ZNB_AMI."SET FIELD X" ("Command") MEDIDA_cRIO_ZNB_AMI."SET FIELD Y" ("Command") MEDIDA_cRIO_ZNB_AMI."SET FIELD Z" ("Command") MEDIDA_cRIO_ZNB_AMI."MEASURE PARAMETERS" ("Command")] -> w122
              frame -1, Default {
              }
              frame 0 {
              }
              frame 1 {
              }
              frame 2 {
              }
              frame 3 {
              }
            }
            n38 = call "Time Delay4"("error in (no error)"=w115, "Delay Time (s)"=0.0) -> ("error out"=w114:errorcluster)  [unwired: 9 in]
            n39 = Greater Or Equal?(x=w108, y=w109) -> (x >= y?=w129:bool)
            n40 = Select(t=w122, s=w129, f=MEDIDA_cRIO_ZNB_AMI."FINALIZAR" ("Command")) -> (s? t:f=w128:T3)
            n41 = local write "cRIO Stable"(FALSE ("PPMS Stable")) -> ()
          }
          frame "SET FIELD X" {
            # "SET FIELD"
            # "Extrae el nuevo valor del campo"
            n42 = global read "cRIO_ZNB_AMI_GLOBALES.vi" "TotalSequence"() -> (w149:string[])
            n43 = Index Array(array=w149, index=w163) -> (element=w148:string)
            n44 = call "Display_Module.vi"("Command"=Display_Command_Control."Generate Event", "error in (no error)"=w151, "Data"="Estableciendo nuevo campo X..." ("element"), "Data Type"=DataType."Update Status") -> ("error out"=w150:errorcluster)  [unwired: 7 in]
            n45 = call "AMI_String_Field X.vi"("String"=w148) -> ("X Rate"=w144:dbl, "X Field"=w143:dbl, "X H.Wait Stability"=w145:bool, "X Modo Rampa"=w139:u16)  [unwired: 6 in, 1 out]
            n46 = local write "X Rate"(w144) -> ()
            n47 = local write "X Field"(w143) -> ()
            n48 = call "elapsedStepMinutesModule.vi"("Command"=Timing_Module_Control."Initialize Time", "error in (no error)"=w150) -> ("error out"=w142:errorcluster)  [unwired: 7 in, 2 out]
            n49 = flat-sequence {
              tunnel: w143 -> [w165]
              tunnel: w144 -> [w166]
              tunnel: w142 -> [_]
              tunnel: w139 -> [w164]
              frame #0 {
                n50 = global write "cRIO_ZNB_AMI_GLOBALES.vi" "rampingMode X"(w164) -> ()
                n51 = global write "cRIO_ZNB_AMI_GLOBALES.vi" "Target X(T)"(w165) -> ()
                n52 = global write "cRIO_ZNB_AMI_GLOBALES.vi" "Rate X(T/min)"(w166) -> ()
              }
              frame #1 {
                # "Set Campo y Rate"
                n53 = global write "cRIO_ZNB_AMI_GLOBALES.vi" "Remote SET X"(TRUE ("TRemoteChange")) -> ()
              }
              frame #2 {
                n54 = call "Time Delay7"("Delay Time (s)"=0.25) -> ()  [unwired: 10 in, 1 out]
              }
              frame #3 {
                # "Start RAMP"
                n55 = global write "cRIO_ZNB_AMI_GLOBALES.vi" "Remote RAMP X"(TRUE ("TRemoteChange")) -> ()
              }
            }
            n56 = local write "X Modo Rampa"(w139) -> ()
            n57 = global write "cRIO_ZNB_AMI_GLOBALES.vi" "X Stable"(FALSE ("V Stable")) -> ()
            n58 = local write "X.Stable"(FALSE ("PPMS Stable")) -> ()
            n59 = Not(x=w145) -> (.not. x?=w138:bool)
            n60 = Select(t=MEDIDA_cRIO_ZNB_AMI."TEST COMMAND" ("Command"), s=w138, f=MEDIDA_cRIO_ZNB_AMI."LOOK STABLE FIELD X" ("Command")) -> (s? t:f=w140:T3)
            n61 = call "Time Delay8"("error in (no error)"=w142, "Delay Time (s)"=5.0) -> ("error out"=w159:errorcluster)  [unwired: 9 in]
          }
          frame "LOOK STABLE FIELD X" {
            # "WAIT STABLE"
            # "Esperaremos a que campo se estabilice sin medir \ny luego seguimos con el siguiente comando"
            # "If NOT stable for a long time\nCONTINUE"
            n62 = call "Time Delay5"("error in (no error)"=w193, "Delay Time (s)"=0.25) -> ("error out"=w192:errorcluster)  [unwired: 9 in]
            n63 = Number To Fractional String(number=w187, precision (6)=i16 1) -> (F-format string=w191:string)  [unwired: 2 in]
            n64 = global read "cRIO_ZNB_AMI_GLOBALES.vi" "Temperature Status"() -> (w186:i32)
            n65 = Concatenate Strings("Esperando campo X estable.... " ("element"), w191) -> (w188:string)
            n66 = global read "cRIO_ZNB_AMI_GLOBALES.vi" "X state"() -> (w201:T1)
            n67 = global read "cRIO_ZNB_AMI_GLOBALES.vi" "Y state"() -> (w173:T1)
            n68 = global read "cRIO_ZNB_AMI_GLOBALES.vi" "Z state"() -> (w172:T1)
            n69 = call "Display_Module.vi"("Command"=Display_Command_Control."Generate Event", "error in (no error)"=w192, "Data"=w188, "Data Type"=DataType."Update Status") -> ("error out"=w181:errorcluster)  [unwired: 7 in]
            n70 = local write "Temperature Status"(w186) -> ()
            n71 = local write "X state"(w201) -> ()
            n72 = local write "Y state"(w173) -> ()
            n73 = local write "Z state"(w172) -> ()
            n74 = call "elapsedTotalMinutesModule.vi"("Command"=Timing_Module_Control."Check Time", "error in (no error)"=w181) -> ("error out"=w180:errorcluster, "Elapsed Out"=w179:dbl)  [unwired: 7 in, 1 out]
            n75 = shared-variable "NI-cRIO9074-PEPA\\Mod1\\AI1"() -> (w175:dbl)  [unwired: 1 in, 1 out]
            n76 = global read "cRIO_ZNB_AMI_GLOBALES.vi" "X field (T)"() -> (w171:dbl)
            n77 = global read "cRIO_ZNB_AMI_GLOBALES.vi" "Y field (T)"() -> (w170:dbl)
            n78 = global read "cRIO_ZNB_AMI_GLOBALES.vi" "Z field (T)"() -> (w184:dbl)
            n79 = global read "cRIO_ZNB_AMI_GLOBALES.vi" "Temperatura(K)"() -> (w183:dbl)
            n80 = shared-variable "NI-cRIO9074-PEPA\\Mod1\\AI2"() -> (w176:dbl)  [unwired: 1 in, 1 out]
            n81 = shared-variable "NI-cRIO9074-PEPA\\Mod1\\AI3"() -> (w177:dbl)  [unwired: 1 in, 1 out]
            n82 = Bundle By Name(cluster=w203, "CampoX(T)"=w171, "CampoY(T)"=w170, "CampoZ(T)"=w184, "Temperatura(K)"=w183, "Tiempo(min)"=w179, "A.Input2(V)"=w175, "A.Input3(V)"=w176, "A.Input4(V)"=w177) -> (w202:T4)
            n83 = local read "StabilityTimeout(s)"() -> (w200:dbl)
            n84 = call "Time Delay3"("error in (no error)"=w180, "Delay Time (s)"=0.0) -> ("error out"=w185:errorcluster)  [unwired: 9 in]
            n85 = To Double Precision Float(number=w200) -> (double precision float=w198:dbl)
            n86 = global read "cRIO_ZNB_AMI_GLOBALES.vi" "X ramping"() -> (w174:bool)
            n87 = Divide(x=w198, y=60.0) -> (x/y=w197:dbl)
            n88 = Not(x=w174) -> (.not. x?=w196:bool)
            n89 = call "elapsedStepMinutesModule.vi"("Command"=Timing_Module_Control."Check Time", "error in (no error)"=w185, "Time In"=w197) -> ("error out"=w204:errorcluster)  [unwired: 6 in, 2 out]
            n90 = Select(t=MEDIDA_cRIO_ZNB_AMI."TEST COMMAND" ("Command"), s=w196, f=MEDIDA_cRIO_ZNB_AMI."LOOK STABLE FIELD X" ("Command")) -> (s? t:f=w208:T3)
            n91 = call "Display_Module.vi"("Command"=Display_Command_Control."Generate Event", "error in (no error)"=w204, "Data"=w202, "Data Type"=DataType."Update Graph") -> ("error out"=w195:errorcluster)  [unwired: 7 in]
          }
          frame "SET FIELD Y" {
            # "SET FIELD"
            # "Extrae el nuevo valor del campo"
            n92 = global read "cRIO_ZNB_AMI_GLOBALES.vi" "TotalSequence"() -> (w228:string[])
            n93 = Index Array(array=w228, index=w242) -> (element=w227:string)
            n94 = call "Display_Module.vi"("Command"=Display_Command_Control."Generate Event", "error in (no error)"=w230, "Data"="Estableciendo nuevo campo Y ..." ("element"), "Data Type"=DataType."Update Status") -> ("error out"=w229:errorcluster)  [unwired: 7 in]
            n95 = call "AMI_String_Field Y.vi"("String"=w227) -> ("Y Rate"=w223:dbl, "Y Field"=w222:dbl, "Y H.Wait Stability"=w224:bool, "Y Modo Rampa"=w218:u16)  [unwired: 6 in, 1 out]
            n96 = local write "Y Rate"(w223) -> ()
            n97 = local write "Y Field"(w222) -> ()
            n98 = call "elapsedStepMinutesModule.vi"("Command"=Timing_Module_Control."Initialize Time", "error in (no error)"=w229) -> ("error out"=w221:errorcluster)  [unwired: 7 in, 2 out]
            n99 = flat-sequence {
              tunnel: w222 -> [w244]
              tunnel: w223 -> [w245]
              tunnel: w221 -> [_]
              tunnel: w218 -> [w243]
              frame #0 {
                n100 = global write "cRIO_ZNB_AMI_GLOBALES.vi" "rampingMode Y"(w243) -> ()
                n101 = global write "cRIO_ZNB_AMI_GLOBALES.vi" "Target Y(T)"(w244) -> ()
                n102 = global write "cRIO_ZNB_AMI_GLOBALES.vi" "Rate Y(T/min)"(w245) -> ()
              }
              frame #1 {
                # "Set Campo y Rate"
                n103 = global write "cRIO_ZNB_AMI_GLOBALES.vi" "Remote SET Y"(TRUE ("TRemoteChange")) -> ()
              }
              frame #2 {
                n104 = call "Time Delay11"("Delay Time (s)"=0.25) -> ()  [unwired: 10 in, 1 out]
              }
              frame #3 {
                # "Start RAMP"
                n105 = global write "cRIO_ZNB_AMI_GLOBALES.vi" "Remote RAMP Y"(TRUE ("TRemoteChange")) -> ()
              }
            }
            n106 = local write "Y Modo Rampa"(w218) -> ()
            n107 = global write "cRIO_ZNB_AMI_GLOBALES.vi" "Y Stable"(FALSE ("V Stable")) -> ()
            n108 = local write "Y.Stable"(FALSE ("PPMS Stable")) -> ()
            n109 = Not(x=w224) -> (.not. x?=w217:bool)
            n110 = Select(t=MEDIDA_cRIO_ZNB_AMI."TEST COMMAND" ("Command"), s=w217, f=MEDIDA_cRIO_ZNB_AMI."LOOK STABLE FIELD Y" ("Command")) -> (s? t:f=w219:T3)
            n111 = call "Time Delay2"("error in (no error)"=w221, "Delay Time (s)"=5.0) -> ("error out"=w238:errorcluster)  [unwired: 9 in]
          }
          frame "LOOK STABLE FIELD Y" {
            # "WAIT STABLE"
            # "Esperaremos a que campo se estabilice sin medir \ny luego seguimos con el siguiente comando"
            # "If NOT stable for a long time\nCONTINUE"
            n112 = call "Time Delay13"("error in (no error)"=w272, "Delay Time (s)"=0.25) -> ("error out"=w271:errorcluster)  [unwired: 9 in]
            n113 = Number To Fractional String(number=w266, precision (6)=i16 1) -> (F-format string=w270:string)  [unwired: 2 in]
            n114 = global read "cRIO_ZNB_AMI_GLOBALES.vi" "Temperature Status"() -> (w265:i32)
            n115 = Concatenate Strings("Esperando campo Y estable.... " ("element"), w270) -> (w267:string)
            n116 = global read "cRIO_ZNB_AMI_GLOBALES.vi" "X state"() -> (w280:T1)
            n117 = global read "cRIO_ZNB_AMI_GLOBALES.vi" "Y state"() -> (w252:T1)
            n118 = global read "cRIO_ZNB_AMI_GLOBALES.vi" "Z state"() -> (w251:T1)
            n119 = call "Display_Module.vi"("Command"=Display_Command_Control."Generate Event", "error in (no error)"=w271, "Data"=w267, "Data Type"=DataType."Update Status") -> ("error out"=w260:errorcluster)  [unwired: 7 in]
            n120 = local write "Temperature Status"(w265) -> ()
            n121 = local write "X state"(w280) -> ()
            n122 = local write "Y state"(w252) -> ()
            n123 = local write "Z state"(w251) -> ()
            n124 = call "elapsedTotalMinutesModule.vi"("Command"=Timing_Module_Control."Check Time", "error in (no error)"=w260) -> ("error out"=w259:errorcluster, "Elapsed Out"=w258:dbl)  [unwired: 7 in, 1 out]
            n125 = shared-variable "NI-cRIO9074-PEPA\\Mod1\\AI1"() -> (w254:dbl)  [unwired: 1 in, 1 out]
            n126 = global read "cRIO_ZNB_AMI_GLOBALES.vi" "X field (T)"() -> (w250:dbl)
            n127 = global read "cRIO_ZNB_AMI_GLOBALES.vi" "Y field (T)"() -> (w249:dbl)
            n128 = global read "cRIO_ZNB_AMI_GLOBALES.vi" "Z field (T)"() -> (w263:dbl)
            n129 = global read "cRIO_ZNB_AMI_GLOBALES.vi" "Temperatura(K)"() -> (w262:dbl)
            n130 = shared-variable "NI-cRIO9074-PEPA\\Mod1\\AI2"() -> (w255:dbl)  [unwired: 1 in, 1 out]
            n131 = shared-variable "NI-cRIO9074-PEPA\\Mod1\\AI3"() -> (w256:dbl)  [unwired: 1 in, 1 out]
            n132 = Bundle By Name(cluster=w282, "CampoX(T)"=w250, "CampoY(T)"=w249, "CampoZ(T)"=w263, "Temperatura(K)"=w262, "Tiempo(min)"=w258, "A.Input2(V)"=w254, "A.Input3(V)"=w255, "A.Input4(V)"=w256) -> (w281:T4)
            n133 = local read "StabilityTimeout(s)"() -> (w279:dbl)
            n134 = call "Time Delay12"("error in (no error)"=w259, "Delay Time (s)"=0.0) -> ("error out"=w264:errorcluster)  [unwired: 9 in]
            n135 = To Double Precision Float(number=w279) -> (double precision float=w277:dbl)
            n136 = global read "cRIO_ZNB_AMI_GLOBALES.vi" "Y ramping"() -> (w253:bool)
            n137 = Divide(x=w277, y=60.0) -> (x/y=w276:dbl)
            n138 = Not(x=w253) -> (.not. x?=w275:bool)
            n139 = call "elapsedStepMinutesModule.vi"("Command"=Timing_Module_Control."Check Time", "error in (no error)"=w264, "Time In"=w276) -> ("error out"=w283:errorcluster)  [unwired: 6 in, 2 out]
            n140 = Select(t=MEDIDA_cRIO_ZNB_AMI."TEST COMMAND" ("Command"), s=w275, f=MEDIDA_cRIO_ZNB_AMI."LOOK STABLE FIELD Y" ("Command")) -> (s? t:f=w287:T3)
            n141 = call "Display_Module.vi"("Command"=Display_Command_Control."Generate Event", "error in (no error)"=w283, "Data"=w281, "Data Type"=DataType."Update Graph") -> ("error out"=w274:errorcluster)  [unwired: 7 in]
          }
          frame "SET FIELD Z" {
            # "SET FIELD"
            # "Extrae el nuevo valor del campo"
            n142 = global read "cRIO_ZNB_AMI_GLOBALES.vi" "TotalSequence"() -> (w307:string[])
            n143 = Index Array(array=w307, index=w321) -> (element=w306:string)
            n144 = call "Display_Module.vi"("Command"=Display_Command_Control."Generate Event", "error in (no error)"=w309, "Data"="Estableciendo nuevo campo Z ..." ("element"), "Data Type"=DataType."Update Status") -> ("error out"=w308:errorcluster)  [unwired: 7 in]
            n145 = call "AMI_String_Field Z.vi"("String"=w306) -> ("Z Rate"=w302:dbl, "Z Field"=w301:dbl, "Z H.Wait Stability"=w303:bool, "Z Modo Rampa"=w297:u16)  [unwired: 6 in, 1 out]
            n146 = local write "Z Rate"(w302) -> ()
            n147 = local write "Z Field"(w301) -> ()
            n148 = call "elapsedStepMinutesModule.vi"("Command"=Timing_Module_Control."Initialize Time", "error in (no error)"=w308) -> ("error out"=w300:errorcluster)  [unwired: 7 in, 2 out]
            n149 = flat-sequence {
              tunnel: w301 -> [w323]
              tunnel: w302 -> [w324]
              tunnel: w300 -> [_]
              tunnel: w297 -> [w322]
              frame #0 {
                n150 = global write "cRIO_ZNB_AMI_GLOBALES.vi" "rampingMode Z"(w322) -> ()
                n151 = global write "cRIO_ZNB_AMI_GLOBALES.vi" "Target Z(T)"(w323) -> ()
                n152 = global write "cRIO_ZNB_AMI_GLOBALES.vi" "Rate Z(T/min)"(w324) -> ()
              }
              frame #1 {
                # "Set Campo y Rate"
                n153 = global write "cRIO_ZNB_AMI_GLOBALES.vi" "Remote SET Z"(TRUE ("TRemoteChange")) -> ()
              }
              frame #2 {
                n154 = call "Time Delay19"("Delay Time (s)"=0.25) -> ()  [unwired: 10 in, 1 out]
              }
              frame #3 {
                # "Start RAMP"
                n155 = global write "cRIO_ZNB_AMI_GLOBALES.vi" "Remote RAMP Z"(TRUE ("TRemoteChange")) -> ()
              }
            }
            n156 = local write "Z Modo Rampa"(w297) -> ()
            n157 = global write "cRIO_ZNB_AMI_GLOBALES.vi" "Z Stable"(FALSE ("V Stable")) -> ()
            n158 = local write "Z.Stable"(FALSE ("PPMS Stable")) -> ()
            n159 = Not(x=w303) -> (.not. x?=w296:bool)
            n160 = Select(t=MEDIDA_cRIO_ZNB_AMI."TEST COMMAND" ("Command"), s=w296, f=MEDIDA_cRIO_ZNB_AMI."LOOK STABLE FIELD Z" ("Command")) -> (s? t:f=w298:T3)
            n161 = call "Time Delay17"("error in (no error)"=w300, "Delay Time (s)"=5.0) -> ("error out"=w317:errorcluster)  [unwired: 9 in]
          }
          frame "LOOK STABLE FIELD Z" {
            # "WAIT STABLE"
            # "Esperaremos a que campo se estabilice sin medir \ny luego seguimos con el siguiente comando"
            # "If NOT stable for a long time\nCONTINUE"
            n162 = call "Time Delay21"("error in (no error)"=w351, "Delay Time (s)"=0.25) -> ("error out"=w350:errorcluster)  [unwired: 9 in]
            n163 = Number To Fractional String(number=w345, precision (6)=i16 1) -> (F-format string=w349:string)  [unwired: 2 in]
            n164 = global read "cRIO_ZNB_AMI_GLOBALES.vi" "Temperature Status"() -> (w344:i32)
            n165 = Concatenate Strings("Esperando campo Z estable.... " ("element"), w349) -> (w346:string)
            n166 = global read "cRIO_ZNB_AMI_GLOBALES.vi" "X state"() -> (w359:T1)
            n167 = global read "cRIO_ZNB_AMI_GLOBALES.vi" "Y state"() -> (w331:T1)
            n168 = global read "cRIO_ZNB_AMI_GLOBALES.vi" "Z state"() -> (w330:T1)
            n169 = call "Display_Module.vi"("Command"=Display_Command_Control."Generate Event", "error in (no error)"=w350, "Data"=w346, "Data Type"=DataType."Update Status") -> ("error out"=w339:errorcluster)  [unwired: 7 in]
            n170 = local write "Temperature Status"(w344) -> ()
            n171 = local write "X state"(w359) -> ()
            n172 = local write "Y state"(w331) -> ()
            n173 = local write "Z state"(w330) -> ()
            n174 = call "elapsedTotalMinutesModule.vi"("Command"=Timing_Module_Control."Check Time", "error in (no error)"=w339) -> ("error out"=w338:errorcluster, "Elapsed Out"=w337:dbl)  [unwired: 7 in, 1 out]
            n175 = shared-variable "NI-cRIO9074-PEPA\\Mod1\\AI1"() -> (w333:dbl)  [unwired: 1 in, 1 out]
            n176 = global read "cRIO_ZNB_AMI_GLOBALES.vi" "X field (T)"() -> (w329:dbl)
            n177 = global read "cRIO_ZNB_AMI_GLOBALES.vi" "Y field (T)"() -> (w328:dbl)
            n178 = global read "cRIO_ZNB_AMI_GLOBALES.vi" "Z field (T)"() -> (w342:dbl)
            n179 = global read "cRIO_ZNB_AMI_GLOBALES.vi" "Temperatura(K)"() -> (w341:dbl)
            n180 = shared-variable "NI-cRIO9074-PEPA\\Mod1\\AI2"() -> (w334:dbl)  [unwired: 1 in, 1 out]
            n181 = shared-variable "NI-cRIO9074-PEPA\\Mod1\\AI3"() -> (w335:dbl)  [unwired: 1 in, 1 out]
            n182 = Bundle By Name(cluster=w361, "CampoX(T)"=w329, "CampoY(T)"=w328, "CampoZ(T)"=w342, "Temperatura(K)"=w341, "Tiempo(min)"=w337, "A.Input2(V)"=w333, "A.Input3(V)"=w334, "A.Input4(V)"=w335) -> (w360:T4)
            n183 = local read "StabilityTimeout(s)"() -> (w358:dbl)
            n184 = call "Time Delay20"("error in (no error)"=w338, "Delay Time (s)"=0.0) -> ("error out"=w343:errorcluster)  [unwired: 9 in]
            n185 = To Double Precision Float(number=w358) -> (double precision float=w356:dbl)
            n186 = global read "cRIO_ZNB_AMI_GLOBALES.vi" "Z ramping"() -> (w332:bool)
            n187 = Divide(x=w356, y=60.0) -> (x/y=w355:dbl)
            n188 = Not(x=w332) -> (.not. x?=w354:bool)
            n189 = call "elapsedStepMinutesModule.vi"("Command"=Timing_Module_Control."Check Time", "error in (no error)"=w343, "Time In"=w355) -> ("error out"=w362:errorcluster)  [unwired: 6 in, 2 out]
            n190 = Select(t=MEDIDA_cRIO_ZNB_AMI."TEST COMMAND" ("Command"), s=w354, f=MEDIDA_cRIO_ZNB_AMI."LOOK STABLE FIELD Z" ("Command")) -> (s? t:f=w366:T3)
            n191 = call "Display_Module.vi"("Command"=Display_Command_Control."Generate Event", "error in (no error)"=w362, "Data"=w360, "Data Type"=DataType."Update Graph") -> ("error out"=w353:errorcluster)  [unwired: 7 in]
          }
          frame "SET TEMPERATURE" {
            w375 = MEDIDA_cRIO_ZNB_AMI."LOOK STABLE TEMPERATURE" ("Command")
            # "Al medir con analizador de frecuencia ENA3G\nsiempre será FALSE. Ira primero a estabilizar, antes de ir a medir"
            # "Set Temperatura 4.2K at 20K/min, FastSettle, Sweep&meas"
            # "Set Temperatura 4.2K at 20K/min, FastSettle, Wait"
            # "SET TEMPERATURA"
            # "Obtiene los parámetros siguientes:  Nueva temperatura\n\nSi se programa sweep mediremos en continuo hasta que temperatura sea estable\nSi NO hay sweep, esperaremos a que temperatura se estabilice sin medir"
            # "Set Temperatura 100K at 1K/min, FastSettle, Sweep and meas"
            # "Extrae el nuevo valor de la tempertura"
            n192 = global read "cRIO_ZNB_AMI_GLOBALES.vi" "TotalSequence"() -> (w384:string[])
            n193 = Index Array(array=w384, index=w397) -> (element=w383:string)
            n194 = call "String_Temperature.vi"("String"=w383) -> ("Rate"=w377:dbl, "Temperature"=w378:dbl, "T.Wait Stability"=w381:bool)  [unwired: 7 in, 1 out]
            "T.WaitStability" <- w381
            n195 = call "Display_Module.vi"("Command"=Display_Command_Control."Generate Event", "error in (no error)"=w386, "Data"="Estableciendo nueva temperatura..." ("element"), "Data Type"=DataType."Update Status") -> ("error out"=w385:errorcluster)  [unwired: 7 in]
            n196 = call "elapsedStepMinutesModule.vi"("Command"=Timing_Module_Control."Initialize Time", "error in (no error)"=w385) -> ("error out"=w379:errorcluster)  [unwired: 7 in, 2 out]
            n197 = flat-sequence {
              tunnel: w378 -> [w400]
              tunnel: w377 -> [w399]
              frame #0 {
                n198 = global write "cRIO_ZNB_AMI_GLOBALES.vi" "Rate(K/min)"(w399) -> ()
                n199 = global write "cRIO_ZNB_AMI_GLOBALES.vi" "SetpointT(K)"(w400) -> ()
                n200 = global write "cRIO_ZNB_AMI_GLOBALES.vi" "TRemoteChange"(TRUE ("TRemoteChange")) -> ()
              }
            }
            n201 = global write "cRIO_ZNB_AMI_GLOBALES.vi" "T Stable"(FALSE ("V Stable")) -> ()
            n202 = local write "T.Stable"(FALSE ("PPMS Stable")) -> ()
            n203 = Select(t=MEDIDA_cRIO_ZNB_AMI."MEASURE SWEEP" ("Command"), s=w381, f=w375) -> ()  [unwired: 1 out]
            n204 = call "Time Delay14"("error in (no error)"=w379, "Delay Time (s)"=1.0) -> ("error out"=w394:errorcluster)  [unwired: 9 in]
          }
          frame "LOOK STABLE TEMPERATURE" {
            # "WAIT STABLE"
            # "Esperaremos a que temperatura se estabilice sin medir \ny luego seguimos con el siguiente comando"
            # "If NOT stable for a long time\nCONTINUE"
            n205 = call "Time Delay16"("error in (no error)"=w426, "Delay Time (s)"=0.25) -> ("error out"=w425:errorcluster)  [unwired: 9 in]
            n206 = Number To Fractional String(number=w419, precision (6)=i16 2) -> (F-format string=w422:string)  [unwired: 2 in]
            n207 = Concatenate Strings("Esperando temperatura estable... " ("element"), w422) -> (w420:string)
            n208 = call "Display_Module.vi"("Command"=Display_Command_Control."Generate Event", "error in (no error)"=w425, "Data"=w420, "Data Type"=DataType."Update Status") -> ("error out"=w416:errorcluster)  [unwired: 7 in]
            n209 = global read "cRIO_ZNB_AMI_GLOBALES.vi" "Temperature Status"() -> (w407:i32)
            n210 = global read "cRIO_ZNB_AMI_GLOBALES.vi" "X state"() -> (w408:T1)
            n211 = global read "cRIO_ZNB_AMI_GLOBALES.vi" "Y state"() -> (w406:T1)
            n212 = global read "cRIO_ZNB_AMI_GLOBALES.vi" "Z state"() -> (w405:T1)
            n213 = local write "Temperature Status"(w407) -> ()
            n214 = local write "X state"(w408) -> ()
            n215 = local write "Y state"(w406) -> ()
            n216 = local write "Z state"(w405) -> ()
            n217 = call "elapsedTotalMinutesModule.vi"("Command"=Timing_Module_Control."Check Time", "error in (no error)"=w416) -> ("error out"=w415:errorcluster, "Elapsed Out"=w414:dbl)  [unwired: 7 in, 1 out]
            n218 = shared-variable "NI-cRIO9074-PEPA\\Mod1\\AI1"() -> (w410:dbl)  [unwired: 1 in, 1 out]
            n219 = shared-variable "NI-cRIO9074-PEPA\\Mod1\\AI2"() -> (w412:dbl)  [unwired: 1 in, 1 out]
            n220 = global read "cRIO_ZNB_AMI_GLOBALES.vi" "X field (T)"() -> (w401:dbl)
            n221 = global read "cRIO_ZNB_AMI_GLOBALES.vi" "Y field (T)"() -> (w402:dbl)
            n222 = global read "cRIO_ZNB_AMI_GLOBALES.vi" "Z field (T)"() -> (w403:dbl)
            n223 = global read "cRIO_ZNB_AMI_GLOBALES.vi" "Temperatura(K)"() -> (w404:dbl)
            n224 = shared-variable "NI-cRIO9074-PEPA\\Mod1\\AI3"() -> (w411:dbl)  [unwired: 1 in, 1 out]
            n225 = Bundle By Name(cluster=w434, "CampoX(T)"=w401, "CampoY(T)"=w402, "CampoZ(T)"=w403, "Temperatura(K)"=w404, "Tiempo(min)"=w414, "A.Input2(V)"=w410, "A.Input3(V)"=w412, "A.Input4(V)"=w411) -> (w433:T4)
            n226 = local read "StabilityTimeout(s)"() -> (w432:dbl)
            n227 = global read "cRIO_ZNB_AMI_GLOBALES.vi" "T Stable"() -> (w409:bool)
            n228 = call "Time Delay18"("error in (no error)"=w415, "Delay Time (s)"=0.0) -> ("error out"=w418:errorcluster)  [unwired: 9 in]
            n229 = To Double Precision Float(number=w432) -> (double precision float=w430:dbl)
            n230 = local write "T.Stable"(w409) -> ()
            n231 = Divide(x=w430, y=60.0) -> (x/y=w429:dbl)
            n232 = call "elapsedStepMinutesModule.vi"("Command"=Timing_Module_Control."Check Time", "error in (no error)"=w418, "Time In"=w429) -> ("error out"=w435:errorcluster)  [unwired: 6 in, 2 out]
            n233 = Or(x=w409, y=w409) -> (x .or. y?=w428:bool)
            n234 = Select(t=MEDIDA_cRIO_ZNB_AMI."TEST COMMAND" ("Command"), s=w428, f=MEDIDA_cRIO_ZNB_AMI."LOOK STABLE TEMPERATURE" ("Command")) -> (s? t:f=w439:T3)
            n235 = call "Display_Module.vi"("Command"=Display_Command_Control."Generate Event", "error in (no error)"=w435, "Data"=w433, "Data Type"=DataType."Update Graph") -> ("error out"=w424:errorcluster)  [unwired: 7 in]
          }
          frame "SET VOLTAGE" {
            w448 = MEDIDA_cRIO_ZNB_AMI."LOOK STABLE VOLTAGE" ("Command")
            # "Al medir con analizador de frecuencia ENA3G\nno se ejecutará nunca esta ventana"
            # "Set Voltage 4.2V at 20V/min, Sweep&meas"
            # "Set Voltage 4.2V at 20V/min, Wait"
            # "SET TEMPERATURA"
            # "Obtiene los parámetros siguientes:  Nueva temperatura\n\nSi se programa sweep mediremos en continuo hasta que temperatura sea estable\nSi NO hay sweep, esperaremos a que temperatura se estabilice sin medir"
            n236 = global read "cRIO_ZNB_AMI_GLOBALES.vi" "TotalSequence"() -> (w457:string[])
            n237 = Index Array(array=w457, index=w470) -> (element=w456:string)
            n238 = call "String_Voltage.vi"("String"=w456) -> ("Rate"=w450:dbl, "Voltage"=w451:dbl, "V.Wait Stability"=w454:bool)  [unwired: 8 in]
            "V.WaitStability" <- w454
            n239 = call "Display_Module.vi"("Command"=Display_Command_Control."Generate Event", "error in (no error)"=w459, "Data"="Estableciendo nuevo voltaje..." ("element"), "Data Type"=DataType."Update Status") -> ("error out"=w458:errorcluster)  [unwired: 7 in]
            n240 = call "elapsedStepMinutesModule.vi"("Command"=Timing_Module_Control."Initialize Time", "error in (no error)"=w458) -> ("error out"=w452:errorcluster)  [unwired: 7 in, 2 out]
            n241 = flat-sequence {
              tunnel: w451 -> [w473]
              tunnel: w450 -> [w472]
              frame #0 {
                n242 = global write "cRIO_ZNB_AMI_GLOBALES.vi" "Rate(V/min)"(w472) -> ()
                n243 = global write "cRIO_ZNB_AMI_GLOBALES.vi" "SetpointV(V)"(w473) -> ()
                n244 = global write "cRIO_ZNB_AMI_GLOBALES.vi" "VRemoteChange"(TRUE ("TRemoteChange")) -> ()
              }
            }
            n245 = global write "cRIO_ZNB_AMI_GLOBALES.vi" "V Stable"(FALSE ("V Stable")) -> ()
            n246 = local write "T.Stable"(FALSE ("PPMS Stable")) -> ()
            n247 = Select(t=MEDIDA_cRIO_ZNB_AMI."MEASURE SWEEP" ("Command"), s=w454, f=w448) -> ()  [unwired: 1 out]
            n248 = call "Time Delay"("error in (no error)"=w452, "Delay Time (s)"=0.0) -> ("error out"=w467:errorcluster)  [unwired: 9 in]
          }
          frame "LOOK STABLE VOLTAGE" {
            # "WAIT STABLE"
            # "Esperaremos a que temperatura se estabilice sin medir \ny luego seguimos con el siguiente comando"
            # "If NOT stable for a long time\nCONTINUE"
            n249 = call "Time Delay10"("error in (no error)"=w499, "Delay Time (s)"=0.25) -> ("error out"=w498:errorcluster)  [unwired: 9 in]
            n250 = Number To Fractional String(number=w492, precision (6)=i16 2) -> (F-format string=w495:string)  [unwired: 2 in]
            n251 = Concatenate Strings("Esperando voltaje estable... " ("element"), w495) -> (w493:string)
            n252 = call "Display_Module.vi"("Command"=Display_Command_Control."Generate Event", "error in (no error)"=w498, "Data"=w493, "Data Type"=DataType."Update Status") -> ("error out"=w487:errorcluster)  [unwired: 7 in]
            n253 = global read "cRIO_ZNB_AMI_GLOBALES.vi" "Temperature Status"() -> (w478:i32)
            n254 = global read "cRIO_ZNB_AMI_GLOBALES.vi" "X state"() -> (w479:T1)
            n255 = global read "cRIO_ZNB_AMI_GLOBALES.vi" "Y state"() -> (w477:T1)
            n256 = global read "cRIO_ZNB_AMI_GLOBALES.vi" "Z state"() -> (w476:T1)
            n257 = call "elapsedTotalMinutesModule.vi"("Command"=Timing_Module_Control."Check Time", "error in (no error)"=w487) -> ("error out"=w486:errorcluster, "Elapsed Out"=w485:dbl)  [unwired: 7 in, 1 out]
            n258 = local write "Temperature Status"(w478) -> ()
            n259 = local write "X state"(w479) -> ()
            n260 = local write "Y state"(w477) -> ()
            n261 = local write "Z state"(w476) -> ()
            n262 = shared-variable "NI-cRIO9074-PEPA\\Mod1\\AI1"() -> (w481:dbl)  [unwired: 1 in, 1 out]
            n263 = global read "cRIO_ZNB_AMI_GLOBALES.vi" "X field (T)"() -> (w474:dbl)
            n264 = global read "cRIO_ZNB_AMI_GLOBALES.vi" "Y field (T)"() -> (w475:dbl)
            n265 = global read "cRIO_ZNB_AMI_GLOBALES.vi" "Z field (T)"() -> (w489:dbl)
            n266 = global read "cRIO_ZNB_AMI_GLOBALES.vi" "Temperatura(K)"() -> (w490:dbl)
            n267 = shared-variable "NI-cRIO9074-PEPA\\Mod1\\AI2"() -> (w482:dbl)  [unwired: 1 in, 1 out]
            n268 = shared-variable "NI-cRIO9074-PEPA\\Mod1\\AI3"() -> (w483:dbl)  [unwired: 1 in, 1 out]
            n269 = Bundle By Name(cluster=w507, "CampoX(T)"=w474, "CampoY(T)"=w475, "CampoZ(T)"=w489, "Temperatura(K)"=w490, "Tiempo(min)"=w485, "A.Input2(V)"=w481, "A.Input3(V)"=w482, "A.Input4(V)"=w483) -> (w506:T4)
            n270 = local read "StabilityTimeout(s)"() -> (w505:dbl)
            n271 = global read "cRIO_ZNB_AMI_GLOBALES.vi" "V Stable"() -> (w480:bool)
            n272 = call "Time Delay9"("error in (no error)"=w486, "Delay Time (s)"=0.0) -> ("error out"=w491:errorcluster)  [unwired: 9 in]
            n273 = To Double Precision Float(number=w505) -> (double precision float=w503:dbl)
            n274 = local write "V.Stable"(w480) -> ()
            n275 = Divide(x=w503, y=60.0) -> (x/y=w502:dbl)
            n276 = call "elapsedStepMinutesModule.vi"("Command"=Timing_Module_Control."Check Time", "error in (no error)"=w491, "Time In"=w502) -> ("error out"=w508:errorcluster)  [unwired: 6 in, 2 out]
            n277 = Or(x=w480, y=w480) -> (x .or. y?=w501:bool)
            n278 = Select(t=MEDIDA_cRIO_ZNB_AMI."TEST COMMAND" ("Command"), s=w501, f=MEDIDA_cRIO_ZNB_AMI."LOOK STABLE VOLTAGE" ("Command")) -> (s? t:f=w512:T3)
            n279 = call "Display_Module.vi"("Command"=Display_Command_Control."Generate Event", "error in (no error)"=w508, "Data"=w506, "Data Type"=DataType."Update Graph") -> ("error out"=w497:errorcluster)  [unwired: 7 in]
          }
          frame "WAIT PARAMETERS" {
            # "Obtiene los parámetros siguientes:\n\n- Esperar a Temperatura estable ?\n- Esperar a Campo estable ?\n-Tiempo maximo de espera de estabilidad\n- Que hacemos si no estabiliza ?"
            # "Wait for Temperature, Timeout 300sec, Continue"
            n280 = global read "cRIO_ZNB_AMI_GLOBALES.vi" "TotalSequence"() -> (w528:string[])
            n281 = Index Array(array=w528, index=w535) -> (element=w527:string)
            n282 = call "String_Wait.vi"("String"=w527) -> ("On timeout"=w521:i32, "Timeout(s)"=w522:i16, "Temperature"=w523:bool)  [unwired: 7 in, 1 out]
            n283 = local write "wT.Stable"(w523) -> ()
            n284 = local write "On timeout"(w521) -> ()
            n285 = local write "StabilityTimeout(s)"(w522) -> ()
            n286 = call "Time Delay15"("error in (no error)"=w524, "Delay Time (s)"=0.25) -> ("error out"=w531:errorcluster)  [unwired: 9 in]
          }
          frame "MEASURE PARAMETERS" {
            # "Extrae los parámetros de medida del VNA"
            # "MEDIDA CON ANALIZADOR DE FRECUENCIA RS ZNB"
            # "Spectrum from 1.0E+5 Hz to 1.0E+6 Hz, Bandwidth 25.00 Hz, 201 points, Power -20.00 dB"
            # "Si #seconds NO es 0 --> estamos en modo sweep&meas"
            # "Si #seconds SI es 0 --> estamos en modo scan"
            # "Obtiene los parámetros siguientes:"
            n287 = global read "cRIO_ZNB_AMI_GLOBALES.vi" "TotalSequence"() -> (w545:string[])
            n288 = Index Array(array=w545, index=w552) -> (element=w544:string)
            n289 = call "String_ENA3G Parameters.vi"("String"=w544) -> ("MeasConfig"=→"MeasConfig":T2)  [unwired: 9 in, 1 out]
            n290 = Equal To 0?(x=0.0) -> (x = 0?=w541:bool)
            n291 = Select(t=MEDIDA_cRIO_ZNB_AMI."SCAN READ TIME, B y T" ("Command"), s=w541, f=MEDIDA_cRIO_ZNB_AMI."TEST COMMAND" ("Command")) -> ()  [unwired: 1 out]
            n292 = call "Time Delay6"("error in (no error)"=w542, "Delay Time (s)"=0.25) -> ("error out"=w548:errorcluster)  [unwired: 9 in]
          }
          frame "MEASURE ENA3G / ZNB" {
            # "MEDIDA CON ANALIZADOR DE FRECUENCIA ZNB"
            # "antes: MEDIDA CON ANALIZADOR DE FRECUENCIA ENA3G"
            n293 = local read "currentPoint"() -> (w575:i16)
            n294 = Increment(x=w575) -> (x+1=w574:i16)
            n295 = local write "currentPoint"(w574) -> ()
            n296 = global read "cRIO_ZNB_AMI_GLOBALES.vi" "Temperature Status"() -> (w561:i32)
            n297 = global read "cRIO_ZNB_AMI_GLOBALES.vi" "X state"() -> (w562:T1)
            n298 = global read "cRIO_ZNB_AMI_GLOBALES.vi" "Y state"() -> (w560:T1)
            n299 = global read "cRIO_ZNB_AMI_GLOBALES.vi" "Z state"() -> (w559:T1)
            n300 = call "Display_Module.vi"("Command"=Display_Command_Control."Generate Event", "error in (no error)"=w577, "Data"="Leyendo T, B", "Data Type"=DataType."Update Status") -> ("error out"=w576:errorcluster)  [unwired: 7 in]
            n301 = global read "cRIO_ZNB_AMI_GLOBALES.vi" "Temperatura(K)"() -> (w566:dbl)
            n302 = global read "cRIO_ZNB_AMI_GLOBALES.vi" "X field (T)"() -> (w553:dbl)
            n303 = global read "cRIO_ZNB_AMI_GLOBALES.vi" "Y field (T)"() -> (w554:dbl)
            n304 = global read "cRIO_ZNB_AMI_GLOBALES.vi" "Z field (T)"() -> (w555:dbl)
            n305 = local write "Temperature Status"(w561) -> ()
            n306 = local write "X state"(w562) -> ()
            n307 = local write "Y state"(w560) -> ()
            n308 = local write "Z state"(w559) -> ()
            n309 = call "elapsedTotalMinutesModule.vi"("Command"=Timing_Module_Control."Check Time", "error in (no error)"=w576) -> ("error out"=w569:errorcluster, "Elapsed Out"=w556:dbl)  [unwired: 7 in, 1 out]
            n310 = local read "MeasConfig"() -> (w570:T2)
            n311 = Bundle By Name(cluster=w570, "Tiempo (sec)"=w556, "Campo X (T)"=w553, "Campo Y (T)"=w554, "Campo Z (T)"=w555, "Temperatura (K)"=w566) -> (w567:T2)
            n312 = local read "ENA3G path"() -> (w565:path)
            n313 = local read "VISA resource"() -> (w564:refnum<visa-resource-name>)
            n314 = local write "MeasConfig"(w567) -> ()
            n315 = call "RohdeSchwarz ZNB ReadSpectrum.vi"("Fichero"=w565, "error in (no error)"=w569, "MeasConfig"=w567, "visa VNA"=w564) -> ("error out"=w568:errorcluster, "XY Graph"=w563:cluster{dbl[], dbl[]})  [unwired: 6 in]
            "XY lastMeas" <- w563
            n316 = global write "cRIO_ZNB_AMI_GLOBALES.vi" "ENA3G Config"(w567) -> ()
            n317 = global write "cRIO_ZNB_AMI_GLOBALES.vi" "XY Graph"(w563) -> ()
            n318 = global read "cRIO_ZNB_AMI_GLOBALES.vi" "X field (T)"() -> (w558:dbl)
            n319 = global read "cRIO_ZNB_AMI_GLOBALES.vi" "Y field (T)"() -> (w557:dbl)
            n320 = global read "cRIO_ZNB_AMI_GLOBALES.vi" "Z field (T)"() -> (w573:dbl)
            n321 = global read "cRIO_ZNB_AMI_GLOBALES.vi" "Temperatura(K)"() -> (w572:dbl)
            n322 = Bundle By Name(cluster=w587, "Tiempo(min)"=w556, "CampoX(T)"=w558, "CampoY(T)"=w557, "CampoZ(T)"=w573, "Temperatura(K)"=w572) -> (w586:T4)
          }
          frame "FINALIZAR" {
            n323 = call "Display_Module.vi"("Command"=Display_Command_Control."Generate Event", "error in (no error)"=w589, "Data"="Fin de programa", "Data Type"=DataType."Update Status") -> ("error out"=w594:errorcluster)  [unwired: 7 in]
            n324 = call "Display_Module.vi"("Command"=Display_Command_Control."Generate Event", "error in (no error)"=w594, "Data"=0, "Data Type"=DataType."Update Front Panel") -> ("error out"=w590:errorcluster)  [unwired: 7 in]
          }
        }
        "Datos" <- w23
        "Command" <- w31
        n325 = local write "error out"(w20) -> ()
        n326 = call "cRIO_ZNB_AMI_STOP.vi"("error in (no error)"=w20, "Stop"=enum16{"Continue", "Stop", "Default"}."Default") -> ("error out"=w34:errorcluster, "Stop?"=w33:bool)  [unwired: 8 in]
        n327 = Or(x=w33, y=w37) -> (x .or. y?=w38:bool)
      }
    }
    frame Error {
    }
  }
  n328 = call "Display_Module.vi"("Command"=Display_Command_Control."Generate Event", "error in (no error)"=w6, "Data"="Fin de programa", "Data Type"=DataType."Update Status") -> ("error out"=w11:errorcluster)  [unwired: 7 in]
  n329 = call "Display_Module.vi"("Command"=Display_Command_Control."Generate Event", "error in (no error)"=w11, "Data"=0, "Data Type"=DataType."Enable/Disable Controls") -> ("error out"=w4:errorcluster)  [unwired: 7 in]
  n330 = call "cRIO_ZNB_AMI_STOP.vi"("error in (no error)"=w4, "Stop"=enum16{"Continue", "Stop", "Default"}."Continue") -> ("error out"=→"error out":errorcluster)  [unwired: 8 in, 1 out]
